vi "Tower_Crane_Balance_Monitor.vi"() -> ()   [LabVIEW 2018]
uses:
  <vilib>/Utility/error.llb/DialogType.ctl
panel:
  out "new picture 4":picture caption="Opertion_Guide"
  out "new picture 3":picture caption="Opertion_Guide"
  out "new picture 2":picture caption="Opertion_Guide"
  out "stanard_section 2":picture caption="配平状态"
  out "X倾斜角度 2":dbl caption="塔身X倾斜角度" format="%#_3g"
  out "Y倾斜角度  2":dbl caption="塔身Y倾斜角度" format="%#_3g"
  out "y轴倾角 2":dbl(knob) scale=0.0..5.0
  out "x轴倾角 2":dbl(knob) scale=0.0..5.0
  out "配平指示1":bool
  out "超声波雷达4":dbl format="%.3f"
  out "超声波雷达4 6":dbl(knob) scale=0.0..10.0
  out "超声波雷达35":dbl format="%.3f"
  out "?":dbl(knob) scale=0.0..10.0
  out "超声波雷达2":dbl format="%.3f"
  out "超声波雷达2":dbl(knob) scale=0.0..10.0
  out "超声波雷达1":dbl format="%.3f"
  out "超声波雷达1":dbl(knob) scale=0.0..10.0
  out "起升高度（m）":dbl caption="起升高度（cm）" format="%#_3g"
  out "变幅长度（m）":dbl format="%#_3g"
  out "风速（m/s）":dbl format="%.3f"
  out "Y倾斜角度":dbl caption="套架Y倾斜角度" format="%#_3g"
  out "X倾斜角度":dbl caption="套架X倾斜角度" format="%#_3g"
  out "回转角度（°）":dbl format="%#_3g"
  out "回转角度":dbl(knob) scale=0.0..10.0
  out "风速":dbl(knob) scale=0.0..10.0
  out "变幅长度":dbl(knob) scale=0.0..140.0
  out "y轴倾角":dbl(knob) scale=0.0..5.0
  out "x轴倾角":dbl(knob) scale=0.0..5.0
  out "起升高度":dbl(slide) caption="顶升高度          (cm)" scale=0.0..180.0
  out "section_connect":picture caption="引进节连接"
  out "rotary_support":picture caption="下回转支座"
  out "stanard_section":picture caption="引进节"
  out "pin_shaft":picture caption="爬爪"
  out "jacking_beam":picture caption="顶升横梁"
  out "new picture":picture caption="Opertion_Guide"
  out "引进滑轮":bool
  out "引进节螺栓4":bool
  out "引进节螺栓3":bool
  out "引进节螺栓2":bool
  out "引进节螺栓1":bool
  out "下回转螺栓4":bool
  out "下回转螺栓3":bool
  out "下回转螺栓2":bool
  out "下回转螺栓1":bool
  out "爬爪右侧":bool
  out "爬爪左侧":bool
  out "横梁右侧":bool
  out "横梁左侧":bool
  in  "倾角串口号 2":refnum<visa-resource-name>
  in  "开始配平":bool
  in  "倾角串口号":refnum<visa-resource-name>
  in  "风速串口号":refnum<visa-resource-name>
  in  "回转编码器":refnum<visa-resource-name>
  in  "变幅编码器":refnum<visa-resource-name>
  in  "高度编码器":refnum<visa-resource-name>
  in  "顶升开关":bool
  in  "滚轮直径D":dbl
  out "倾角读取缓冲区 2":string caption="倾角读取缓冲区"
  out "子字符串 4":string
  out "子字符串 3":string
  out "子字符串 2":string
  out "子字符串":string
  out "数据输出 2":string
  out "esp32的IP地址 2":string
  out "信息来源的端口 2":u16
  in  "清空 2":bool
  out "esp32的IP地址":string
  out "回转圈数":dbl
  out "回转编码器读取缓冲区":string
  out "回转单圈值":dbl
  out "回转编码器错误输出":string
  out "变幅圈数":dbl
  out "小车蝙蝠编码器读取缓冲区":string
  out "变幅单圈值":dbl
  out "回转编码器错误输出1":string
  out "倾角读取缓冲区":string
  out "Wind_Speed_Data":string
  out "风速传感器错误输出":string
  out "操作规范":string
  out "起升圈数":dbl
  out "起升高度编码器读取缓冲区 2":string
  out "起升单圈值":dbl
  out "起升高度编码器数值":dbl
  out "高度编码器错误输出1":string
  out "data out":string
  out "数据输出":string
  out "信息来源的端口":u16
  in  "停止":bool
  in  "清空":bool
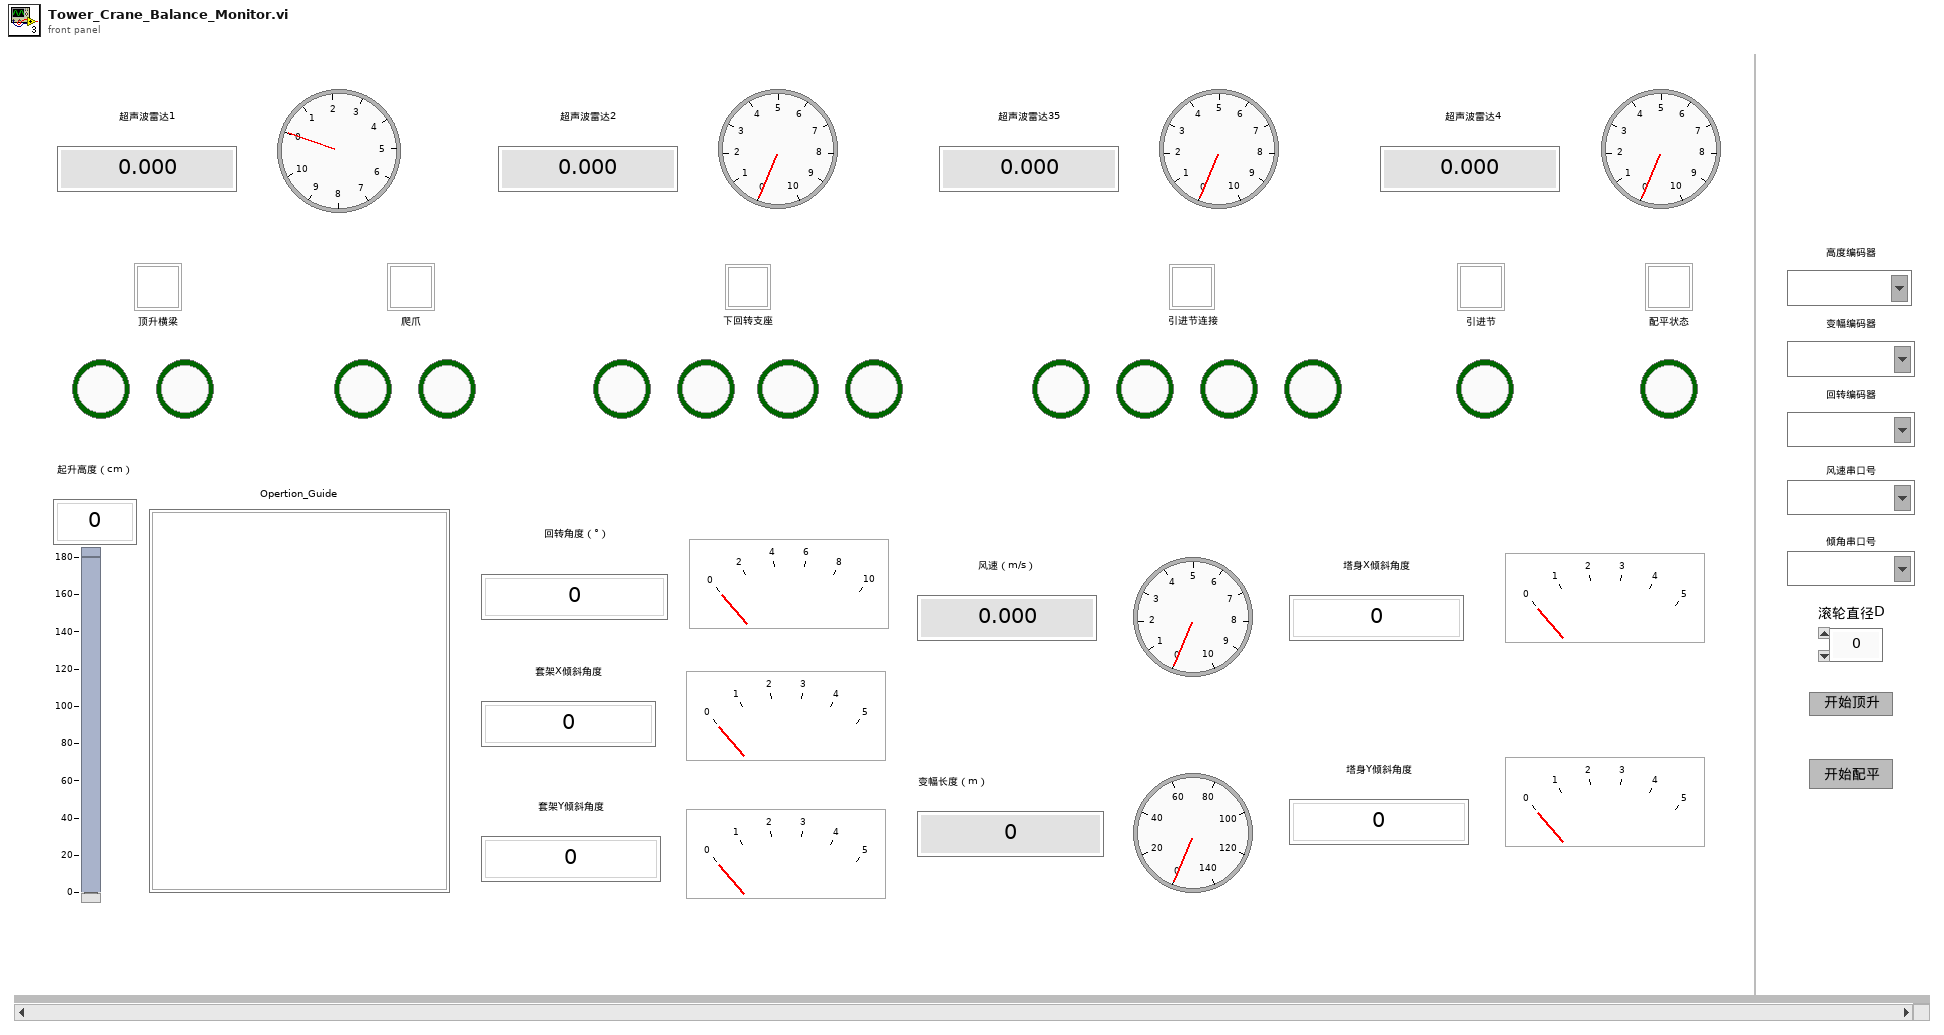
[diagram p1: front panel]
types:
  T1 = typedef "DialogType.ctl" = u16
  T2 = typedef "imagedata.ctl" = cluster{"image type":i32, "image depth":i32, "image":u8[], "mask":u8[], "colors":u32[], "Rectangle":cluster{"left":i16, "top":i16, "right":i16, "bottom":i16}}
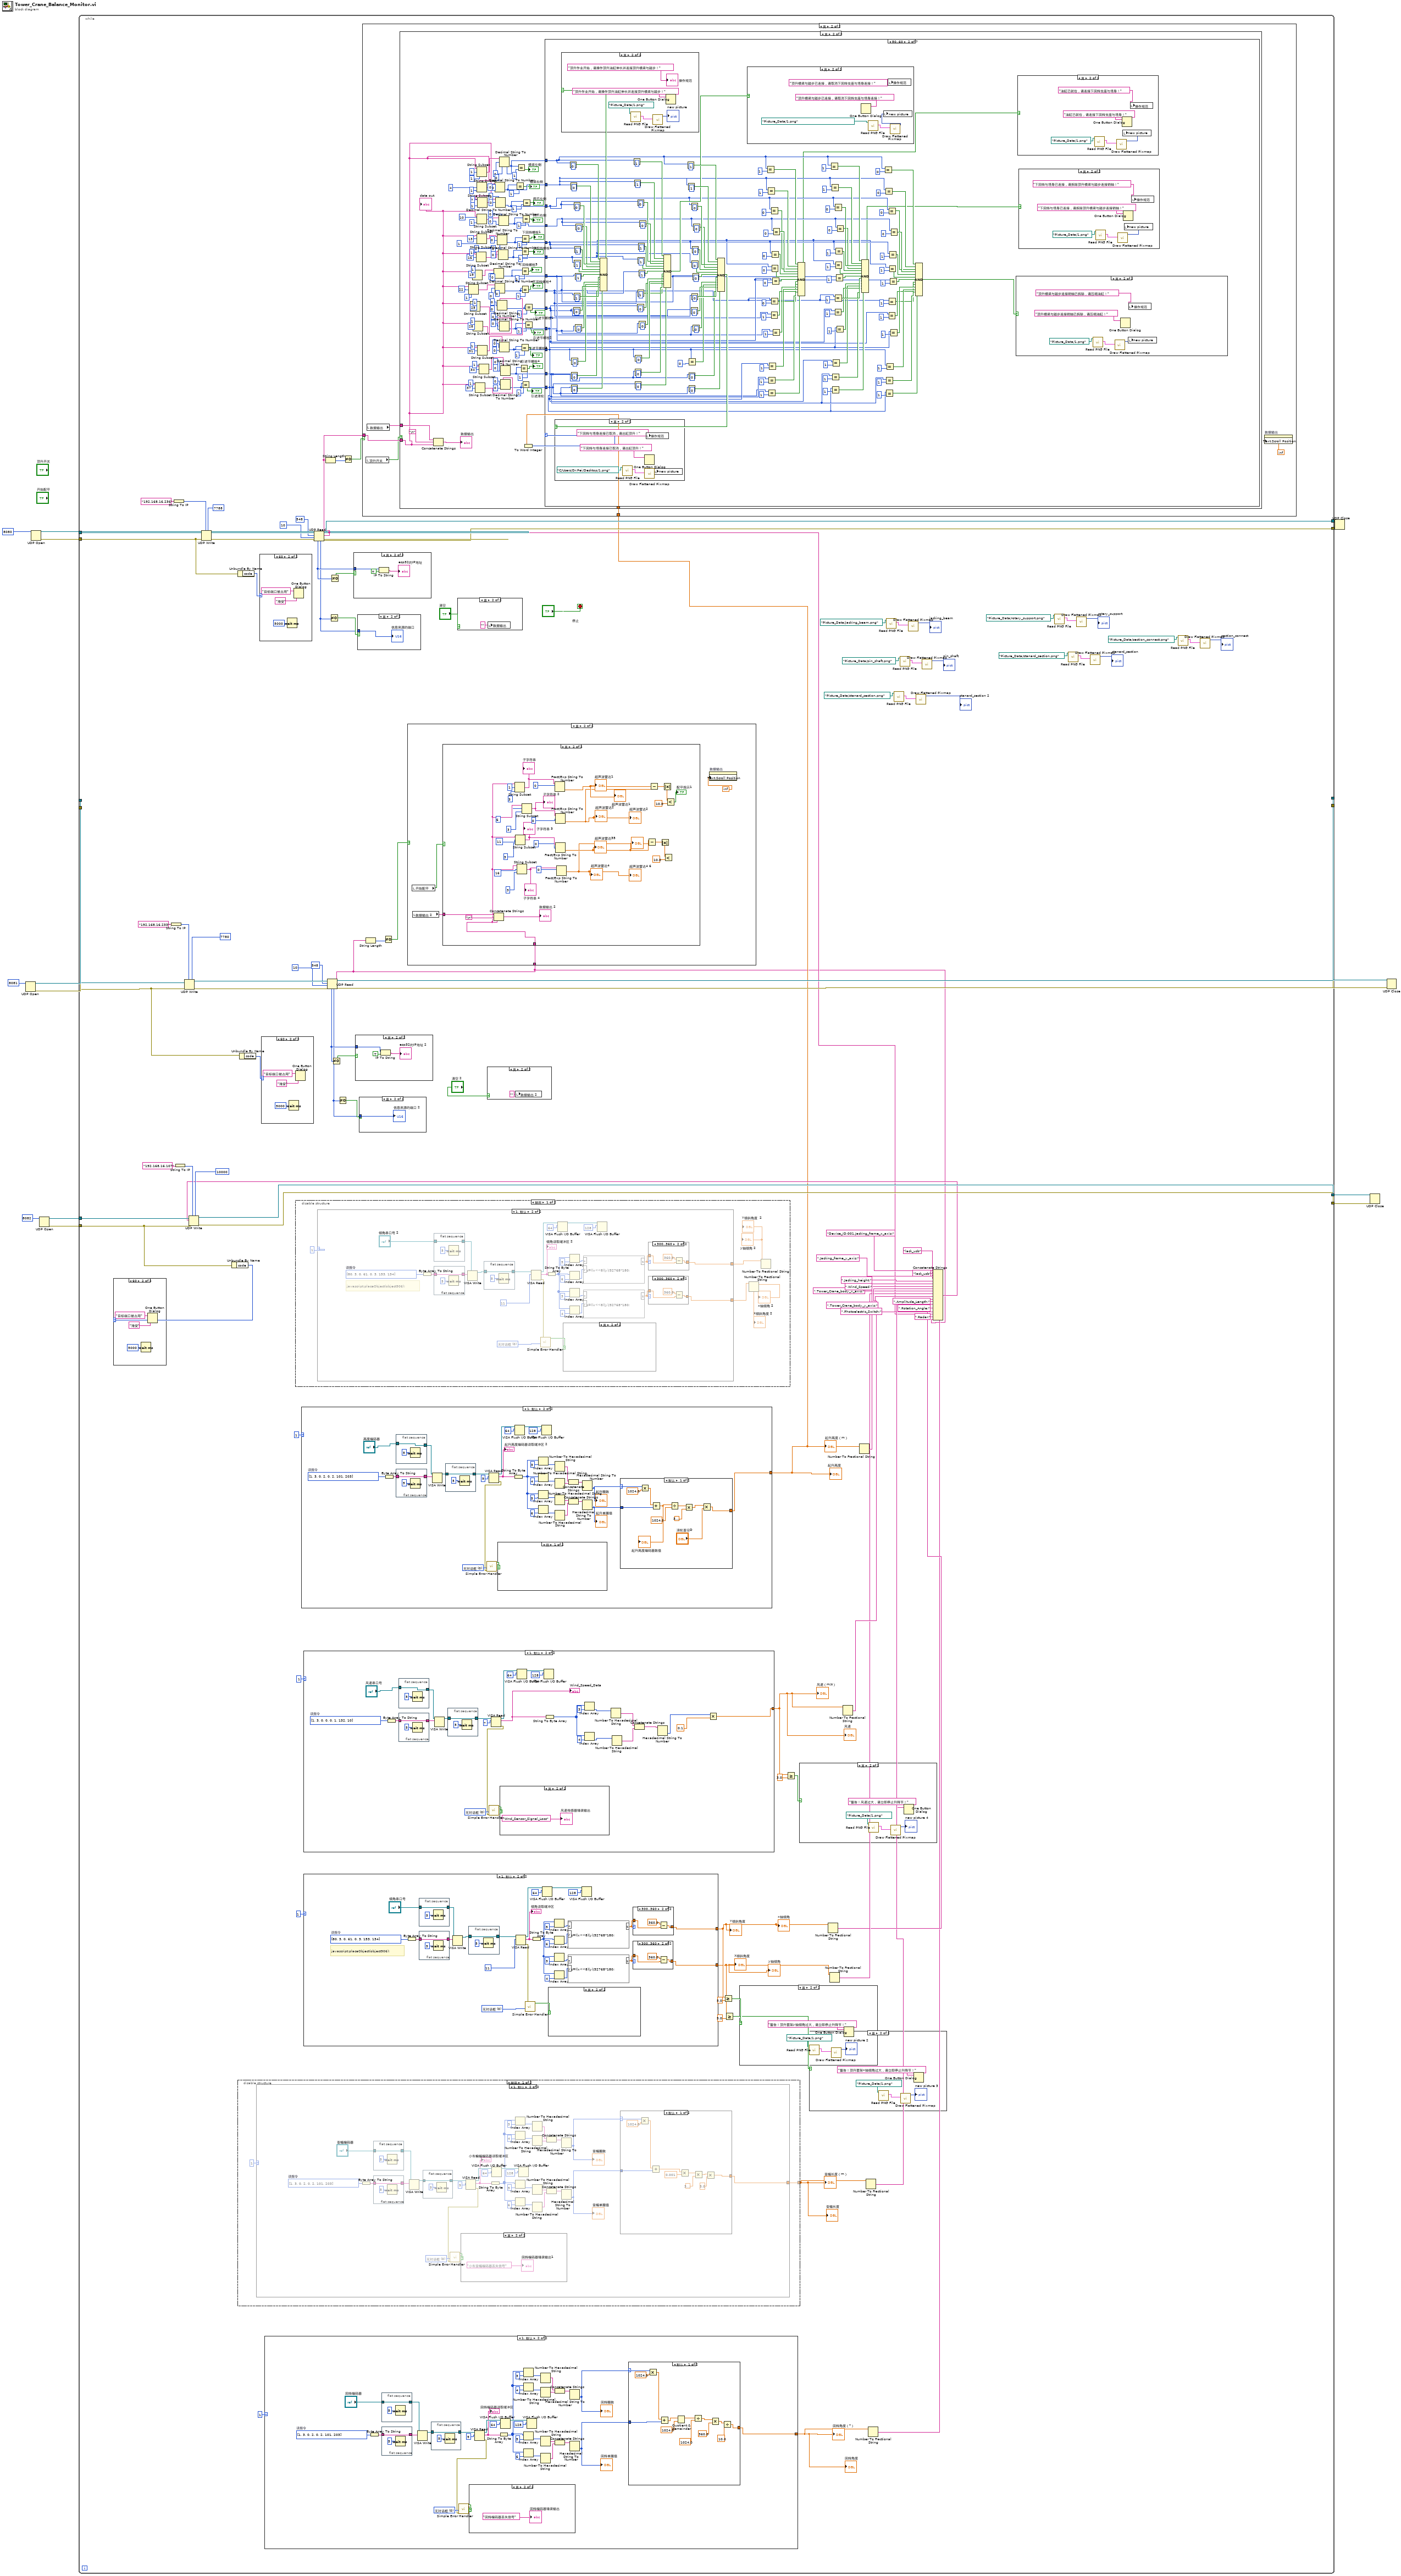
[diagram p0: block diagram]
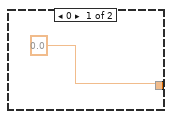
[diagram p2: hidden frame]
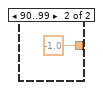
[diagram p4: hidden frame]
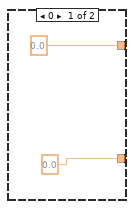
[diagram p9: hidden frame]
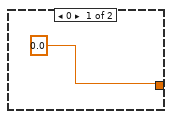
[diagram p14: hidden frame]
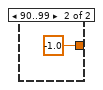
[diagram p16: hidden frame]
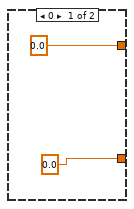
[diagram p17: hidden frame]
diagram:
  n1 = UDP Open(11:u16 8081 ("端口")) -> (port=w9:refnum<k16>, 0:w7:errorcluster)  [unwired: 4 in, 1 out]
  n2 = UDP Open(11:u16 8080 ("端口")) -> (port=w15:refnum<k16>, 0:w14:errorcluster)  [unwired: 4 in, 1 out]
  n3 = UDP Open(11:u16 8082 ("端口")) -> (port=w3:refnum<k16>, 0:w4:errorcluster)  [unwired: 4 in, 1 out]
  n4 = while {
    tunnel: w15 -> [w89]
    tunnel: w14 -> [w84]
    tunnel: [w117] -> w13
    tunnel: [w114] -> w12
    tunnel: w9 -> [w79]
    tunnel: [w77] -> w8
    tunnel: w7 -> [w75]
    tunnel: [w66] -> w6
    tunnel: w4 -> [w58]
    tunnel: w3 -> [w62]
    tunnel: [w57] -> w2
    tunnel: [w56] -> w1
    stop <- "停止" stop-if-true
    n5 = String To IP(1:"192.168.16.233" ("名称")) -> (0:w72:u32)
    n6 = String To IP(1:"192.168.16.236" ("名称")) -> (0:w86:u32)
    n7 = String To IP(1:"192.168.16.107" ("名称")) -> (0:w61:u32)
    n8 = UDP Write(address=w72, port or service name=u16 7780 ("端口或服务名称"), connection ID=w79, 8:w75) -> (error out=w76:errorcluster, 3:w78:refnum<k16>)  [unwired: 2 in]
    n9 = UDP Write(address=w86, port or service name=u16 7788 ("端口或服务名称"), connection ID=w89, 8:w84) -> (error out=w85:errorcluster, 3:w88:refnum<k16>)  [unwired: 2 in]
    n10 = Unbundle By Name(w58) -> ("code"=w59:i32)
    n11 = case shown="60" w59 {
      frame 0, Default {
      }
      frame 60 {
        n12 = Wait (ms)(milliseconds to wait=u32 5000 ("等待时间（毫秒）")) -> ()  [unwired: 1 out]
        n13 = One Button Dialog(message="目标端口被占用" ("消息"), button name ("OK")="难受" ("按钮名称（“确定”）")) -> ()  [unwired: 1 out]
      }
    }
    n14 = disable-structure shown="禁用" {
      disable-tunnel: [w118 _] -> w41
      frame Disabled {
        n15 = case shown="1, 默认" 1 {
          tunnel: [0.0 w126] -> w118
          frame 0 {
          }
          frame 1, Default {
            w124 = T1 0 items=["无对话框", "确定信息", "继续或停止信息", "确定信息＋警告", "继续/停止+警告"] ("type of dialog (OK msg:1)")
            w127 = i32[] [1, 3, 0, 2, 0, 2, 101, 203]  # 读指令
            n16 = Byte Array To String(unsigned byte array=w127) -> (string=w144:string)
            n17 = flat-sequence {
              tunnel: "变幅编码器" -> [w172]
              tunnel: [w172] -> w121
              frame #0 {
                n18 = Wait (ms)(milliseconds to wait=5) -> ()  [unwired: 1 out]
              }
            }
            n19 = flat-sequence {
              tunnel: [w170] -> w143
              tunnel: w144 -> [w170]
              frame #0 {
                n20 = Wait (ms)(milliseconds to wait=5) -> ()  [unwired: 1 out]
              }
            }
            n21 = VISA Write(VISA resource name=w121, write buffer=w143) -> (VISA resource name out=w135:refnum<visa-resource-name>)  [unwired: 1 in, 2 out]
            n22 = flat-sequence {
              tunnel: [w168] -> w136
              tunnel: w135 -> [w168]
              frame #0 {
                n23 = Wait (ms)(milliseconds to wait=5) -> ()  [unwired: 1 out]
              }
            }
            n24 = VISA Read(VISA resource name=w136, byte count=u32 9 ("字节总数")) -> (VISA resource name out=w152:refnum<visa-resource-name>, read buffer=w142:string, error out=w123:errorcluster)  [unwired: 1 in, 1 out]
            "小车蝙蝠编码器读取缓冲区" <- w142
            n25 = call <vilib>:"Simple Error Handler.vi"("type of dialog (OK msg:1)"=w124, "error in (no error)"=w123) -> ("error?"=w125:bool)  [unwired: 3 in, 4 out]
            n26 = case shown="真" w125 {
              frame False {
              }
              frame True {
                "回转编码器错误输出1" <- "小车变幅编码器丢失信号" ("九轴错误输出1")
              }
            }
            n27 = String To Byte Array(string=w142) -> (unsigned byte array=w150:u8[])
            n28 = VISA Flush I/O Buffer(VISA resource name=w152, mask (16)=64) -> (VISA resource name out=w151:refnum<visa-resource-name>)  [unwired: 1 in, 1 out]
            n29 = Index Array ("索引数组")(array=w150, index=3) -> (element=w137:u8)
            n30 = Index Array(array=w150, index=4) -> (element=w141:u8)
            n31 = Index Array ("索引数组")(array=w150, index=5) -> (element=w145:u8)
            n32 = Index Array(array=w150, index=6) -> (element=w149:u8)
            n33 = VISA Flush I/O Buffer(VISA resource name=w151, mask (16)=128) -> ()  [unwired: 1 in, 2 out]
            n34 = Number To Hexadecimal String(2:w137) -> (0:w140:string)  [unwired: 1 in]
            n35 = Number To Hexadecimal String(2:w141) -> (0:w139:string)  [unwired: 1 in]
            n36 = Number To Hexadecimal String(2:w145) -> (0:w148:string)  [unwired: 1 in]
            n37 = Number To Hexadecimal String(2:w149) -> (0:w147:string)  [unwired: 1 in]
            n38 = Concatenate Strings(w140, w139) -> (w138:string)
            n39 = Concatenate Strings(w148, w147) -> (w146:string)
            n40 = Hexadecimal String To Number(string=w138) -> (number=w153:u32)  [unwired: 2 in, 1 out]
            "变幅圈数" <- w153
            n41 = Hexadecimal String To Number(string=w146) -> (number=w154:u32)  [unwired: 2 in, 1 out]
            "变幅单圈值" <- w154
            n42 = case shown="默认" w153 {
              selector: w153 -> [w160 _]
              tunnel: w154 -> [w159 _]
              tunnel: [w158 -1.0] -> w126
              frame Default {
                n43 = Multiply(x=w160, y=1024.0) -> (x*y=w165:dbl)
                n44 = Add(x=w165, y=w159) -> (x+y=w166:dbl)
                n45 = Multiply(x=w166, y=0.001) -> (x*y=w163:dbl)
                n46 = Multiply(x=w163, y=3.141592653589793) -> (x*y=w164:dbl)
                n47 = Multiply(x=w164, y=3.0) -> (x*y=w158:dbl)
              }
              frame 90..99 {
              }
            }
          }
        }
      }
      frame Enabled {
      }
    }
    "变幅长度（m）" <- w41
    "变幅长度" <- w41
    n48 = Unbundle By Name(w84) -> ("code"=w108:i32)
    n49 = Unbundle By Name(w75) -> ("code"=w74:i32)
    n50 = case shown="60" w108 {
      frame 0, Default {
      }
      frame 60 {
        n51 = Wait (ms)(milliseconds to wait=u32 5000 ("等待时间（毫秒）")) -> ()  [unwired: 1 out]
        n52 = One Button Dialog(message="目标端口被占用" ("消息"), button name ("OK")="难受" ("按钮名称（“确定”）")) -> ()  [unwired: 1 out]
      }
    }
    n53 = case shown="60" w74 {
      frame 0, Default {
      }
      frame 60 {
        n54 = Wait (ms)(milliseconds to wait=u32 5000 ("等待时间（毫秒）")) -> ()  [unwired: 1 out]
        n55 = One Button Dialog(message="目标端口被占用" ("消息"), button name ("OK")="难受" ("按钮名称（“确定”）")) -> ()  [unwired: 1 out]
      }
    }
    n56 = case shown="1, 默认" 1 {
      tunnel: [0.0 w240] -> w40
      frame 0 {
      }
      frame 1, Default {
        w238 = T1 0 items=["无对话框", "确定信息", "继续或停止信息", "确定信息＋警告", "继续/停止+警告"] ("type of dialog (OK msg:1)")
        w241 = i32[] [1, 3, 0, 2, 0, 2, 101, 203]  # 读指令
        n57 = Byte Array To String(unsigned byte array=w241) -> (string=w258:string)
        n58 = flat-sequence {
          tunnel: "回转编码器" -> [w288]
          tunnel: [w288] -> w235
          frame #0 {
            n59 = Wait (ms)(milliseconds to wait=5) -> ()  [unwired: 1 out]
          }
        }
        n60 = flat-sequence {
          tunnel: [w286] -> w257
          tunnel: w258 -> [w286]
          frame #0 {
            n61 = Wait (ms)(milliseconds to wait=5) -> ()  [unwired: 1 out]
          }
        }
        n62 = VISA Write(VISA resource name=w235, write buffer=w257) -> (VISA resource name out=w249:refnum<visa-resource-name>)  [unwired: 1 in, 2 out]
        n63 = flat-sequence {
          tunnel: [w284] -> w250
          tunnel: w249 -> [w284]
          frame #0 {
            n64 = Wait (ms)(milliseconds to wait=5) -> ()  [unwired: 1 out]
          }
        }
        n65 = VISA Read(VISA resource name=w250, byte count=u32 9 ("字节总数")) -> (VISA resource name out=w266:refnum<visa-resource-name>, read buffer=w256:string, error out=w237:errorcluster)  [unwired: 1 in, 1 out]
        "回转编码器读取缓冲区" <- w256
        n66 = call <vilib>:"Simple Error Handler.vi"("type of dialog (OK msg:1)"=w238, "error in (no error)"=w237) -> ("error?"=w239:bool)  [unwired: 3 in, 4 out]
        n67 = case shown="真" w239 {
          frame False {
          }
          frame True {
            "回转编码器错误输出" <- "回转编码器丢失信号" ("九轴错误输出1")
          }
        }
        n68 = String To Byte Array(string=w256) -> (unsigned byte array=w264:u8[])
        n69 = VISA Flush I/O Buffer(VISA resource name=w266, mask (16)=64) -> (VISA resource name out=w265:refnum<visa-resource-name>)  [unwired: 1 in, 1 out]
        n70 = Index Array ("索引数组")(array=w264, index=3) -> (element=w251:u8)
        n71 = Index Array(array=w264, index=4) -> (element=w255:u8)
        n72 = Index Array ("索引数组")(array=w264, index=5) -> (element=w259:u8)
        n73 = Index Array(array=w264, index=6) -> (element=w263:u8)
        n74 = VISA Flush I/O Buffer(VISA resource name=w265, mask (16)=128) -> ()  [unwired: 1 in, 2 out]
        n75 = Number To Hexadecimal String(2:w251) -> (0:w254:string)  [unwired: 1 in]
        n76 = Number To Hexadecimal String(2:w255) -> (0:w253:string)  [unwired: 1 in]
        n77 = Number To Hexadecimal String(2:w259) -> (0:w262:string)  [unwired: 1 in]
        n78 = Number To Hexadecimal String(2:w263) -> (0:w261:string)  [unwired: 1 in]
        n79 = Concatenate Strings(w254, w253) -> (w252:string)
        n80 = Concatenate Strings(w262, w261) -> (w260:string)
        n81 = Hexadecimal String To Number(string=w252) -> (number=w267:u32)  [unwired: 2 in, 1 out]
        "回转圈数" <- w267
        n82 = Hexadecimal String To Number(string=w260) -> (number=w268:u32)  [unwired: 2 in, 1 out]
        "回转单圈值" <- w268
        n83 = case shown="默认" w267 {
          selector: w267 -> [w280 _]
          tunnel: w268 -> [w279 _]
          tunnel: [w271 -1.0] -> w240
          frame Default {
            n84 = Multiply(x=w280, y=1024.0) -> (x*y=w282:dbl)
            n85 = Add(x=w282, y=w279) -> (x+y=w278:dbl)
            n86 = Quotient & Remainder(x=w278, y=1024.0) -> (x-y*floor(x/y)=w273:dbl)  [unwired: 1 out]
            n87 = Divide(x=w273, y=1024.0) -> (x/y=w275:dbl)
            n88 = Multiply(x=w275, y=360.0) -> (x*y=w272:dbl)
            n89 = Divide(x=w272, y=10.0) -> (x/y=w271:dbl)
          }
          frame 90..99 {
          }
        }
      }
    }
    "回转角度（°）" <- w40
    "回转角度" <- w40
    n90 = disable-structure shown="禁用" {
      frame Disabled {
        n91 = case shown="1, 默认" 1 {
          tunnel: [0.0 w193] -> w187
          tunnel: [0.0 w199] -> w186
          frame 0 {
          }
          frame 1, Default {
            w196 = T1 0 items=["无对话框", "确定信息", "继续或停止信息", "确定信息＋警告", "继续/停止+警告"] ("type of dialog (OK msg:1)")
            w200 = i32[] [80, 3, 0, 61, 0, 3, 153, 134]  # 读指令
            # "javascript:placeObject(object906);"
            n92 = Byte Array To String(unsigned byte array=w200) -> (string=w212:string)
            n93 = flat-sequence {
              tunnel: "倾角串口号 2" -> [w232]
              tunnel: [w232] -> w194
              frame #0 {
                n94 = Wait (ms)(milliseconds to wait=5) -> ()  [unwired: 1 out]
              }
            }
            n95 = flat-sequence {
              tunnel: [w230] -> w191
              tunnel: w212 -> [w230]
              frame #0 {
                n96 = Wait (ms)(milliseconds to wait=5) -> ()  [unwired: 1 out]
              }
            }
            n97 = VISA Write(VISA resource name=w194, write buffer=w191) -> (VISA resource name out=w208:refnum<visa-resource-name>)  [unwired: 1 in, 2 out]
            n98 = flat-sequence {
              tunnel: w208 -> [w228]
              tunnel: [w228] -> w209
              frame #0 {
                n99 = Wait (ms)(milliseconds to wait=5) -> ()  [unwired: 1 out]
              }
            }
            n100 = VISA Read(VISA resource name=w209, byte count=u32 11 ("字节总数")) -> (VISA resource name out=w216:refnum<visa-resource-name>, read buffer=w192:string, error out=w197:errorcluster)  [unwired: 1 in, 1 out]
            "倾角读取缓冲区 2" <- w192
            n101 = call <vilib>:"Simple Error Handler.vi"("type of dialog (OK msg:1)"=w196, "error in (no error)"=w197) -> ("error?"=w198:bool)  [unwired: 3 in, 4 out]
            n102 = String To Byte Array(string=w192) -> (unsigned byte array=w217:u8[])
            n103 = VISA Flush I/O Buffer(VISA resource name=w216, mask (16)=64) -> (VISA resource name out=w215:refnum<visa-resource-name>)  [unwired: 1 in, 1 out]
            n104 = case shown="真" w198 {
              frame False {
              }
              frame True {
              }
            }
            n105 = Index Array(array=w217, index=5) -> (element=w214:u8)
            n106 = Index Array(array=w217, index=6) -> (element=w213:u8)
            n107 = Index Array(array=w217, index=3) -> (element=w211:u8)
            n108 = Index Array(array=w217, index=4) -> (element=w210:u8)
            n109 = formula code="z=((x<<8)|y)/32768*180;"("x"=w214, "y"=w213) -> ("z"=w219:dbl)
            n110 = formula code="z=((x<<8)|y)/32768*180;"("x"=w211, "y"=w210) -> ("z"=w218:dbl)
            n111 = VISA Flush I/O Buffer(VISA resource name=w215, mask (16)=128) -> ()  [unwired: 1 in, 2 out]
            n112 = case shown="300..360" w219 {
              tunnel: [w224 w226] -> w193
              tunnel: w219 -> [w224 w225]
              frame Default {
              }
              frame 300..360 {
                n113 = Subtract(x=360.0, y=w225) -> (x-y=w226:dbl)
              }
            }
            n114 = case shown="300..360" w218 {
              tunnel: [w220 w222] -> w199
              tunnel: w218 -> [w220 w221]
              frame Default {
              }
              frame 300..360 {
                n115 = Subtract(x=360.0, y=w221) -> (x-y=w222:dbl)
              }
            }
          }
        }
        "X倾斜角度 2" <- w186
        "Y倾斜角度  2" <- w187
        "y轴倾角 2" <- w187
        "x轴倾角 2" <- w186
        n116 = Number To Fractional String(number=w186) -> ()  [unwired: 3 in, 1 out]
        n117 = Number To Fractional String(number=w187) -> ()  [unwired: 3 in, 1 out]
      }
      frame Enabled {
      }
    }
    n118 = case shown="1, 默认" 1 {
      tunnel: [0.0 w376] -> w48
      frame 0 {
      }
      frame 1, Default {
        w374 = T1 0 items=["无对话框", "确定信息", "继续或停止信息", "确定信息＋警告", "继续/停止+警告"] ("type of dialog (OK msg:1)")
        w377 = i32[] [1, 3, 0, 2, 0, 2, 101, 203]  # 读指令
        n119 = Byte Array To String(unsigned byte array=w377) -> (string=w393:string)
        n120 = flat-sequence {
          tunnel: "高度编码器" -> [w422]
          tunnel: [w422] -> w371
          frame #0 {
            n121 = Wait (ms)(milliseconds to wait=5) -> ()  [unwired: 1 out]
          }
        }
        n122 = flat-sequence {
          tunnel: [w420] -> w392
          tunnel: w393 -> [w420]
          frame #0 {
            n123 = Wait (ms)(milliseconds to wait=5) -> ()  [unwired: 1 out]
          }
        }
        n124 = VISA Write(VISA resource name=w371, write buffer=w392) -> (VISA resource name out=w385:refnum<visa-resource-name>)  [unwired: 1 in, 2 out]
        n125 = flat-sequence {
          tunnel: [w418] -> w386
          tunnel: w385 -> [w418]
          frame #0 {
            n126 = Wait (ms)(milliseconds to wait=5) -> ()  [unwired: 1 out]
          }
        }
        n127 = VISA Read(VISA resource name=w386, byte count=u32 9 ("字节总数")) -> (VISA resource name out=w401:refnum<visa-resource-name>, read buffer=w402:string, error out=w373:errorcluster)  [unwired: 1 in, 1 out]
        "起升高度编码器读取缓冲区 2" <- w402
        n128 = call <vilib>:"Simple Error Handler.vi"("type of dialog (OK msg:1)"=w374, "error in (no error)"=w373) -> ("error?"=w375:bool)  [unwired: 3 in, 4 out]
        n129 = case shown="假" w375 {
          frame False {
          }
          frame True {
            "高度编码器错误输出1" <- "起升高度编码器丢失信号" ("九轴错误输出1")
          }
        }
        n130 = String To Byte Array(string=w402) -> (unsigned byte array=w399:u8[])
        n131 = VISA Flush I/O Buffer(VISA resource name=w401, mask (16)=64) -> (VISA resource name out=w400:refnum<visa-resource-name>)  [unwired: 1 in, 1 out]
        n132 = Index Array ("索引数组")(array=w399, index=3) -> (element=w387:u8)
        n133 = Index Array(array=w399, index=4) -> (element=w391:u8)
        n134 = Index Array ("索引数组")(array=w399, index=5) -> (element=w394:u8)
        n135 = Index Array(array=w399, index=6) -> (element=w398:u8)
        n136 = VISA Flush I/O Buffer(VISA resource name=w400, mask (16)=128) -> ()  [unwired: 1 in, 2 out]
        n137 = Number To Hexadecimal String(2:w387) -> (0:w390:string)  [unwired: 1 in]
        n138 = Number To Hexadecimal String(2:w391) -> (0:w389:string)  [unwired: 1 in]
        n139 = Number To Hexadecimal String(2:w394) -> (0:w397:string)  [unwired: 1 in]
        n140 = Number To Hexadecimal String(2:w398) -> (0:w396:string)  [unwired: 1 in]
        n141 = Concatenate Strings(w390, w389) -> (w388:string)
        n142 = Concatenate Strings(w397, w396) -> (w395:string)
        n143 = Hexadecimal String To Number(string=w388) -> (number=w403:u32)  [unwired: 2 in, 1 out]
        "起升圈数" <- w403
        n144 = Hexadecimal String To Number(string=w395) -> (number=w404:u32)  [unwired: 2 in, 1 out]
        "起升单圈值" <- w404
        n145 = case shown="默认" w403 {
          selector: w403 -> [w413 _]
          tunnel: w404 -> [w414 _]
          tunnel: [w406 -1.0] -> w376
          frame Default {
            n146 = Multiply(x=w413, y=1024.0) -> (x*y=w416:dbl)
            n147 = Add(x=w416, y=w414) -> (x+y=w412:dbl)
            "起升高度编码器数值" <- w412
            n148 = Divide(x=w412, y=1024.0) -> (x/y=w410:dbl)
            n149 = Multiply(x=w410, y=3.141592653589793) -> (x*y=w408:dbl)
            n150 = Multiply(x=w408, y="滚轮直径D") -> (x*y=w406:dbl)
          }
          frame 90..99 {
          }
        }
      }
    }
    "起升高度（m）" <- w48
    "起升高度" <- w48
    n151 = case shown="1, 默认" 1 {
      tunnel: [0.0 w298] -> w24
      tunnel: [0.0 w297] -> w22
      frame 0 {
      }
      frame 1, Default {
        w294 = T1 0 items=["无对话框", "确定信息", "继续或停止信息", "确定信息＋警告", "继续/停止+警告"] ("type of dialog (OK msg:1)")
        w299 = i32[] [80, 3, 0, 61, 0, 3, 153, 134]  # 读指令
        # "javascript:placeObject(object906);"
        n152 = Byte Array To String(unsigned byte array=w299) -> (string=w312:string)
        n153 = flat-sequence {
          tunnel: [w333] -> w293
          tunnel: "倾角串口号" -> [w333]
          frame #0 {
            n154 = Wait (ms)(milliseconds to wait=5) -> ()  [unwired: 1 out]
          }
        }
        n155 = flat-sequence {
          tunnel: [w331] -> w313
          tunnel: w312 -> [w331]
          frame #0 {
            n156 = Wait (ms)(milliseconds to wait=5) -> ()  [unwired: 1 out]
          }
        }
        n157 = VISA Write(VISA resource name=w293, write buffer=w313) -> (VISA resource name out=w308:refnum<visa-resource-name>)  [unwired: 1 in, 2 out]
        n158 = flat-sequence {
          tunnel: w308 -> [w329]
          tunnel: [w329] -> w309
          frame #0 {
            n159 = Wait (ms)(milliseconds to wait=5) -> ()  [unwired: 1 out]
          }
        }
        n160 = VISA Read(VISA resource name=w309, byte count=u32 11 ("字节总数")) -> (VISA resource name out=w317:refnum<visa-resource-name>, read buffer=w307:string, error out=w295:errorcluster)  [unwired: 1 in, 1 out]
        "倾角读取缓冲区" <- w307
        n161 = call <vilib>:"Simple Error Handler.vi"("type of dialog (OK msg:1)"=w294, "error in (no error)"=w295) -> ("error?"=w296:bool)  [unwired: 3 in, 4 out]
        n162 = String To Byte Array(string=w307) -> (unsigned byte array=w318:u8[])
        n163 = VISA Flush I/O Buffer(VISA resource name=w317, mask (16)=64) -> (VISA resource name out=w316:refnum<visa-resource-name>)  [unwired: 1 in, 1 out]
        n164 = case shown="真" w296 {
          frame False {
          }
          frame True {
          }
        }
        n165 = Index Array(array=w318, index=5) -> (element=w315:u8)
        n166 = Index Array(array=w318, index=6) -> (element=w314:u8)
        n167 = Index Array(array=w318, index=3) -> (element=w311:u8)
        n168 = Index Array(array=w318, index=4) -> (element=w310:u8)
        n169 = formula code="z=((x<<8)|y)/32768*180;"("x"=w315, "y"=w314) -> ("z"=w320:dbl)
        n170 = formula code="z=((x<<8)|y)/32768*180;"("x"=w311, "y"=w310) -> ("z"=w319:dbl)
        n171 = VISA Flush I/O Buffer(VISA resource name=w316, mask (16)=128) -> ()  [unwired: 1 in, 2 out]
        n172 = case shown="300..360" w320 {
          tunnel: [w325 w327] -> w298
          tunnel: w320 -> [w325 w326]
          frame Default {
          }
          frame 300..360 {
            n173 = Subtract(x=360.0, y=w326) -> (x-y=w327:dbl)
          }
        }
        n174 = case shown="300..360" w319 {
          tunnel: [w321 w323] -> w297
          tunnel: w319 -> [w321 w322]
          frame Default {
          }
          frame 300..360 {
            n175 = Subtract(x=360.0, y=w322) -> (x-y=w323:dbl)
          }
        }
      }
    }
    "X倾斜角度" <- w22
    "Y倾斜角度" <- w24
    "x轴倾角" <- w24
    "y轴倾角" <- w22
    n176 = case shown="1, 默认" 1 {
      tunnel: [u32 0 w337] -> w18
      frame 0 {
      }
      frame 1, Default {
        w351 = T1 0 items=["无对话框", "确定信息", "继续或停止信息", "确定信息＋警告", "继续/停止+警告"] ("type of dialog (OK msg:1)")
        w353 = i32[] [1, 3, 0, 0, 0, 1, 132, 10]  # 读指令
        n177 = Byte Array To String(unsigned byte array=w353) -> (string=w360:string)
        n178 = flat-sequence {
          tunnel: "风速串口号" -> [w368]
          tunnel: [w368] -> w348
          frame #0 {
            n179 = Wait (ms)(milliseconds to wait=5) -> ()  [unwired: 1 out]
          }
        }
        n180 = flat-sequence {
          tunnel: [w366] -> w359
          tunnel: w360 -> [w366]
          frame #0 {
            n181 = Wait (ms)(milliseconds to wait=5) -> ()  [unwired: 1 out]
          }
        }
        n182 = VISA Write(VISA resource name=w348, write buffer=w359) -> (VISA resource name out=w357:refnum<visa-resource-name>)  [unwired: 1 in, 2 out]
        n183 = flat-sequence {
          tunnel: [w364] -> w358
          tunnel: w357 -> [w364]
          frame #0 {
            n184 = Wait (ms)(milliseconds to wait=5) -> ()  [unwired: 1 out]
          }
        }
        n185 = VISA Read(VISA resource name=w358, byte count=u32 7 ("字节总数")) -> (VISA resource name out=w362:refnum<visa-resource-name>, read buffer=w347:string, error out=w350:errorcluster)  [unwired: 1 in, 1 out]
        "Wind_Speed_Data" <- w347
        n186 = call <vilib>:"Simple Error Handler.vi"("type of dialog (OK msg:1)"=w351, "error in (no error)"=w350) -> ("error?"=w352:bool)  [unwired: 3 in, 4 out]
        n187 = case shown="真" w352 {
          frame False {
          }
          frame True {
            "风速传感器错误输出" <- "Wnd_Sensor_Signal_Loss" ("九轴错误输出1")
          }
        }
        n188 = VISA Flush I/O Buffer(VISA resource name=w362, mask (16)=64) -> (VISA resource name out=w361:refnum<visa-resource-name>)  [unwired: 1 in, 1 out]
        n189 = VISA Flush I/O Buffer(VISA resource name=w361, mask (16)=128) -> ()  [unwired: 1 in, 2 out]
        n190 = String To Byte Array(string=w347) -> (unsigned byte array=w346:u8[])
        n191 = Index Array(array=w346, index=3 ("索引")) -> (element=w343:u8)
        n192 = Index Array(array=w346, index=4 ("索引")) -> (element=w342:u8)
        n193 = Number To Hexadecimal String(2:w343) -> (0:w341:string)  [unwired: 1 in]
        n194 = Number To Hexadecimal String(2:w342) -> (0:w340:string)  [unwired: 1 in]
        n195 = Concatenate Strings(w341, w340) -> (w339:string)
        n196 = Hexadecimal String To Number(string=w339) -> (number=w338:u32)  [unwired: 2 in, 1 out]
        n197 = Multiply(x=w338, y=0.1) -> (x*y=w337:dbl)
      }
    }
    "风速" <- w18
    "风速（m/s）" <- w18
    n198 = UDP Read(connection ID=w88, max size (548)=548 ("最大值(548)"), timeout ms (25000)=10 ("超时毫秒(25000)"), 8:w85) -> (data out=w31:string, error out=w117:errorcluster, 3:w114:refnum<k16>, 4:w107:u16, 6:w111:u32)
    n199 = String Length(string=w31) -> (length=w113:i32)
    n200 = UDP Read(connection ID=w78, max size (548)=548 ("最大值(548)"), timeout ms (25000)=10 ("超时毫秒(25000)"), 8:w76) -> (data out=w30:string, error out=w66:errorcluster, 3:w77:refnum<k16>, 4:w67:u16, 6:w68:u32)
    n201 = Not Equal To 0?(x=w107) -> (x != 0?=w109:bool)
    n202 = Not Equal To 0?(x=w111) -> (x != 0?=w110:bool)
    n203 = Not Equal To 0?(x=w68) -> (x != 0?=w80:bool)
    n204 = Not Equal To 0?(x=w67) -> (x != 0?=w81:bool)
    n205 = Not Equal To 0?(x=w113) -> (x != 0?=w112:bool)
    n206 = case shown="真" w110 {
      tunnel: w111 -> [_ w477]
      frame False {
      }
      frame True {
        n207 = IP To String(1:TRUE ("句点符号？(F)"), 2:w477) -> (0:→"esp32的IP地址":string)
      }
    }
    n208 = case shown="真" w80 {
      tunnel: w68 -> [_ w467]
      frame False {
      }
      frame True {
        n209 = IP To String(1:TRUE ("句点符号？(F)"), 2:w467) -> (0:→"esp32的IP地址 2":string)
      }
    }
    n210 = case shown="真" w109 {
      tunnel: w107 -> [_ w474]
      frame False {
      }
      frame True {
        "信息来源的端口" <- w474
      }
    }
    n211 = case shown="真" w81 {
      tunnel: w67 -> [_ w466]
      frame False {
      }
      frame True {
        "信息来源的端口 2" <- w466
      }
    }
    n212 = case shown="真" w112 {
      tunnel: w31 -> [_ w481]
      tunnel: w48 -> [_ w479]
      frame False {
      }
      frame True {
        n213 = local read "顶升开关"() -> (w478:bool)
        n214 = local read "数据输出"() -> (w482:string)
        n215 = case shown="真" w478 {
          tunnel: w482 -> [w485 w594]
          tunnel: w481 -> [w484 w569]
          tunnel: w479 -> [_ w572]
          frame False {
            n216 = Concatenate Strings(w485, w484) -> (w483:string)
            n217 = local write "数据输出"(w483) -> ()
          }
          frame True {
            (unwired) 0 ("默认(0 I32)")
            n218 = Concatenate Strings(w594, "\n", w569) -> (→"数据输出":string)
            n219 = String Subset(string=w569, offset (0)=22 ("偏移量(0)"), length (rest)=1 ("长度（剩余）")) -> (substring=w530:string)
            n220 = String Subset(string=w569, offset (0)=25 ("偏移量(0)"), length (rest)=1 ("长度（剩余）")) -> (substring=w529:string)
            n221 = String Subset(string=w569, offset (0)=19 ("偏移量(0)"), length (rest)=1 ("长度（剩余）")) -> (substring=w531:string)
            n222 = String Subset(string=w569, offset (0)=28 ("偏移量(0)"), length (rest)=1 ("长度（剩余）")) -> (substring=w528:string)
            n223 = String Subset(string=w569, offset (0)=37 ("偏移量(0)"), length (rest)=1 ("长度（剩余）")) -> (substring=w525:string)
            n224 = String Subset(string=w569, offset (0)=16 ("偏移量(0)"), length (rest)=1 ("长度（剩余）")) -> (substring=w547:string)
            n225 = String Subset(string=w569, offset (0)=4 ("偏移量(0)"), length (rest)=1 ("长度（剩余）")) -> (substring=w582:string)
            n226 = String Subset(string=w569, offset (0)=13 ("偏移量(0)"), length (rest)=1 ("长度（剩余）")) -> (substring=w548:string)
            n227 = String Subset(string=w569, offset (0)=1 ("偏移量(0)"), length (rest)=1 ("长度（剩余）")) -> (substring=w584:string)
            n228 = String Subset(string=w569, offset (0)=10 ("偏移量(0)"), length (rest)=1 ("长度（剩余）")) -> (substring=w581:string)
            n229 = String Subset(string=w569, offset (0)=31 ("偏移量(0)"), length (rest)=1 ("长度（剩余）")) -> (substring=w527:string)
            n230 = String Subset(string=w569, offset (0)=7 ("偏移量(0)"), length (rest)=1 ("长度（剩余）")) -> (substring=w583:string)
            n231 = String Subset(string=w569, offset (0)=34 ("偏移量(0)"), length (rest)=1 ("长度（剩余）")) -> (substring=w526:string)
            n232 = Decimal String To Number(string=w531, offset=0 ("偏移量"), default (0L)=0 ("默认(0 I32)")) -> (number=w501:i32)  [unwired: 1 out]
            n233 = Decimal String To Number(string=w582, offset=0 ("偏移量"), default (0L)=0 ("默认(0 I32)")) -> (number=w509:i32)  [unwired: 1 out]
            n234 = Decimal String To Number(string=w530, offset=0 ("偏移量"), default (0L)=0 ("默认(0 I32)")) -> (number=w500:i32)  [unwired: 1 out]
            n235 = Decimal String To Number(string=w583, offset=0 ("偏移量"), default (0L)=0 ("默认(0 I32)")) -> (number=w507:i32)  [unwired: 1 out]
            n236 = Decimal String To Number(string=w548, offset=0 ("偏移量"), default (0L)=0 ("默认(0 I32)")) -> (number=w503:i32)  [unwired: 1 out]
            n237 = Decimal String To Number(string=w529, offset=0 ("偏移量")) -> (number=w499:i32)  [unwired: 1 in, 1 out]
            n238 = Decimal String To Number(string=w547, offset=0 ("偏移量"), default (0L)=0 ("默认(0 I32)")) -> (number=w502:i32)  [unwired: 1 out]
            n239 = Decimal String To Number(string=w581, offset=0 ("偏移量"), default (0L)=0 ("默认(0 I32)")) -> (number=w505:i32)  [unwired: 1 out]
            n240 = Decimal String To Number(string=w584, offset=0 ("偏移量"), default (0L)=0 ("默认(0 I32)")) -> (number=w524:i32)  [unwired: 1 out]
            n241 = Decimal String To Number(string=w528, offset=0 ("偏移量"), default (0L)=0 ("默认(0 I32)")) -> (number=w498:i32)  [unwired: 1 out]
            n242 = Decimal String To Number(string=w527, offset=0 ("偏移量"), default (0L)=0 ("默认(0 I32)")) -> (number=w497:i32)  [unwired: 1 out]
            n243 = Decimal String To Number(string=w526, offset=0 ("偏移量"), default (0L)=0 ("默认(0 I32)")) -> (number=w496:i32)  [unwired: 1 out]
            n244 = Decimal String To Number(string=w525, offset=0 ("偏移量"), default (0L)=0 ("默认(0 I32)")) -> (number=w495:i32)  [unwired: 1 out]
            n245 = Equal?(x=w509, y=1) -> (x = y?=→"横梁右侧":bool)
            n246 = Equal?(x=w524, y=1) -> (x = y?=→"横梁左侧":bool)
            n247 = Equal?(x=w496, y=1) -> (x = y?=→"引进节螺栓4":bool)
            n248 = Equal?(x=w497, y=1) -> (x = y?=→"引进节螺栓3":bool)
            n249 = Equal?(x=w502, y=1) -> (x = y?=→"下回转螺栓2":bool)
            n250 = Equal?(x=w501, y=1) -> (x = y?=→"下回转螺栓3":bool)
            n251 = Equal?(x=w500, y=1) -> (x = y?=→"下回转螺栓4":bool)
            n252 = Equal?(x=w503, y=1) -> (x = y?=→"下回转螺栓1":bool)
            n253 = Equal?(x=w495, y=1) -> (x = y?=→"引进滑轮":bool)
            n254 = Equal?(x=w505, y=1) -> (x = y?=→"爬爪右侧":bool)
            n255 = Equal?(x=w507, y=1) -> (x = y?=→"爬爪左侧":bool)
            n256 = To Word Integer(number=w572) -> (16bit integer=w571:i16)
            n257 = Equal?(x=w498, y=1) -> (x = y?=→"引进节螺栓2":bool)
            n258 = Equal?(x=w499, y=1) -> (x = y?=→"引进节螺栓1":bool)
            n259 = case shown="50..60" w571 {
              tunnel: w524 -> [w610 w725 w940 w1018 w1093 _ w1175]
              tunnel: w509 -> [w609 w724 w941 w1017 w1092 _ w1174]
              tunnel: w507 -> [w608 w723 w939 w1016 w1091 _ w1173]
              tunnel: w505 -> [w607 w722 w938 w1015 w1090 _ w1172]
              tunnel: w503 -> [w606 w721 w937 w1014 w1089 _ w1171]
              tunnel: w502 -> [w605 w720 w936 w1013 w1088 _ w1170]
              tunnel: w501 -> [w604 w719 w935 w1012 w1087 _ w1169]
              tunnel: w500 -> [w603 w718 w934 w1011 w1086 _ w1168]
              tunnel: w499 -> [w602 w717 w933 w1010 w1085 _ w1167]
              tunnel: w498 -> [w601 w710 w932 w1009 w1084 _ w1166]
              tunnel: w497 -> [w600 w716 w931 w1008 w1083 _ w1165]
              tunnel: w496 -> [w599 w715 w930 w1007 w1082 _ w1164]
              tunnel: w495 -> [w598 w714 w929 w1006 w1081 _ w1163]
              frame 25..30, Default {
                n260 = Equal?(x=w610, y=0) -> (x = y?=w688:bool)
                n261 = Equal?(x=w609, y=0) -> (x = y?=w687:bool)
                n262 = Equal?(x=w599, y=0) -> (x = y?=w677:bool)
                n263 = Equal?(x=w598, y=0) -> (x = y?=w676:bool)
                n264 = Equal?(x=w600, y=0) -> (x = y?=w678:bool)
                n265 = Equal?(x=w602, y=0) -> (x = y?=w680:bool)
                n266 = Equal?(x=w608, y=1) -> (x = y?=w686:bool)
                n267 = Equal?(x=w603, y=0) -> (x = y?=w681:bool)
                n268 = Equal?(x=w605, y=0) -> (x = y?=w683:bool)
                n269 = Equal?(x=w606, y=0) -> (x = y?=w684:bool)
                n270 = Equal?(x=w604, y=0) -> (x = y?=w682:bool)
                n271 = Equal?(x=w601, y=0) -> (x = y?=w679:bool)
                n272 = Equal?(x=w607, y=1) -> (x = y?=w685:bool)
                n273 = Compound Arithmetic op=AND ("复合运算")(w688, w687, w686, w685, w684, w683, w682, w681, w680, w679, w678, w677, w676) -> (w597:bool)
                n274 = Equal?(x=w610, y=1) -> (x = y?=w663:bool)
                n275 = Equal?(x=w609, y=1) -> (x = y?=w664:bool)
                n276 = Equal?(x=w599, y=0) -> (x = y?=w674:bool)
                n277 = Equal?(x=w598, y=0) -> (x = y?=w675:bool)
                n278 = Equal?(x=w600, y=0) -> (x = y?=w673:bool)
                n279 = Equal?(x=w602, y=0) -> (x = y?=w671:bool)
                n280 = Equal?(x=w608, y=1) -> (x = y?=w665:bool)
                n281 = Equal?(x=w603, y=0) -> (x = y?=w670:bool)
                n282 = Equal?(x=w605, y=0) -> (x = y?=w668:bool)
                n283 = Equal?(x=w606, y=0) -> (x = y?=w667:bool)
                n284 = Equal?(x=w604, y=0) -> (x = y?=w669:bool)
                n285 = Equal?(x=w601, y=0) -> (x = y?=w672:bool)
                n286 = Equal?(x=w607, y=1) -> (x = y?=w666:bool)
                n287 = Compound Arithmetic op=AND ("复合运算")(w663, w664, w665, w666, w667, w668, w669, w670, w671, w672, w673, w674, w675) -> (w596:bool)
                n288 = Equal?(x=w610, y=1) -> (x = y?=w662:bool)
                n289 = Equal?(x=w609, y=1) -> (x = y?=w661:bool)
                n290 = Equal?(x=w599, y=0) -> (x = y?=w651:bool)
                n291 = Equal?(x=w598, y=0) -> (x = y?=w650:bool)
                n292 = Equal?(x=w600, y=0) -> (x = y?=w652:bool)
                n293 = Equal?(x=w602, y=0) -> (x = y?=w654:bool)
                n294 = Equal?(x=w608, y=0) -> (x = y?=w660:bool)
                n295 = Equal?(x=w603, y=0) -> (x = y?=w655:bool)
                n296 = Equal?(x=w605, y=0) -> (x = y?=w657:bool)
                n297 = Equal?(x=w606, y=0) -> (x = y?=w658:bool)
                n298 = Equal?(x=w604, y=0) -> (x = y?=w656:bool)
                n299 = Equal?(x=w601, y=0) -> (x = y?=w653:bool)
                n300 = Equal?(x=w607, y=0) -> (x = y?=w659:bool)
                n301 = Compound Arithmetic op=AND ("复合运算")(w662, w661, w660, w659, w658, w657, w656, w655, w654, w653, w652, w651, w650) -> (w595:bool)
                n302 = case shown="真" w596 {
                  frame False {
                    n303 = call "Empty Picture"() -> ("empty picture"=w690:picture)
                    n304 = local write "new picture"(w690) -> ()
                    n305 = local write "操作规范"("" ("字符串")) -> ()
                  }
                  frame True {
                    n306 = call <vilib>:"Read PNG File.vi"("path to PNG file"=path "Picture_Data/1.png" ("path to JPEG file")) -> ("image data"=w695:T2)  [unwired: 8 in, 2 out]
                    n307 = call <vilib>:"Draw Flattened Pixmap.vi"("image data"=w695) -> ("new picture"=w691:picture)  [unwired: 8 in]
                    n308 = One Button Dialog(message="顶升横梁与踏步连接销轴已连接，请掀起爬爪！" ("消息")) -> ()  [unwired: 1 in, 1 out]
                    n309 = local write "操作规范"("顶升横梁与踏步连接销轴已连接，请掀起爬爪！" ("字符串")) -> ()
                    n310 = local write "new picture"(w691) -> ()
                  }
                }
                n311 = case shown="真" w597 {
                  frame False {
                    n312 = call "Empty Picture"() -> ("empty picture"=w703:picture)
                    n313 = local write "new picture"(w703) -> ()
                    n314 = local write "操作规范"("" ("字符串")) -> ()
                  }
                  frame True {
                    n315 = call <vilib>:"Read PNG File.vi"("path to PNG file"=path "Picture_Data/1.png" ("path to JPEG file")) -> ("image data"=w709:T2)  [unwired: 8 in, 2 out]
                    n316 = call <vilib>:"Draw Flattened Pixmap.vi"("image data"=w709) -> ("new picture"=w705:picture)  [unwired: 8 in]
                    n317 = One Button Dialog(message="油缸压缩完毕，请连接顶升横梁与踏步连接销轴！" ("消息")) -> ()  [unwired: 1 in, 1 out]
                    n318 = local write "操作规范"("油缸压缩完毕，请连接顶升横梁与踏步连接销轴！" ("字符串")) -> ()
                    n319 = local write "new picture"(w705) -> ()
                  }
                }
                n320 = case shown="真" w595 {
                  frame False {
                    n321 = call "Empty Picture"() -> ("empty picture"=w696:picture)
                    n322 = local write "new picture"(w696) -> ()
                    n323 = local write "操作规范"("" ("字符串")) -> ()
                  }
                  frame True {
                    n324 = call <vilib>:"Read PNG File.vi"("path to PNG file"=path "Picture_Data/1.png" ("path to JPEG file")) -> ("image data"=w702:T2)  [unwired: 8 in, 2 out]
                    n325 = call <vilib>:"Draw Flattened Pixmap.vi"("image data"=w702) -> ("new picture"=w699:picture)  [unwired: 8 in]
                    n326 = local write "操作规范"("爬爪已掀起，请出缸顶升至容纳引进节！" ("字符串")) -> ()
                    n327 = One Button Dialog(message="爬爪已掀起，请出缸顶升至容纳引进节！" ("消息")) -> ()  [unwired: 1 in, 1 out]
                    n328 = local write "new picture"(w699) -> ()
                  }
                }
              }
              frame 50..60 {
                n329 = Equal?(x=w725, y=0) -> (x = y?=w884:bool)
                n330 = Equal?(x=w724, y=0) -> (x = y?=w883:bool)
                n331 = Equal?(x=w715, y=0) -> (x = y?=w873:bool)
                n332 = Equal?(x=w714, y=0) -> (x = y?=w872:bool)
                n333 = Equal?(x=w716, y=0) -> (x = y?=w874:bool)
                n334 = Equal?(x=w717, y=0) -> (x = y?=w876:bool)
                n335 = Equal?(x=w723, y=0) -> (x = y?=w882:bool)
                n336 = Equal?(x=w718, y=1) -> (x = y?=w877:bool)
                n337 = Equal?(x=w720, y=1) -> (x = y?=w879:bool)
                n338 = Equal?(x=w721, y=1) -> (x = y?=w880:bool)
                n339 = Equal?(x=w719, y=1) -> (x = y?=w878:bool)
                n340 = Equal?(x=w710, y=0) -> (x = y?=w875:bool)
                n341 = Equal?(x=w722, y=0) -> (x = y?=w881:bool)
                n342 = Compound Arithmetic op=AND ("复合运算")(w884, w883, w882, w881, w880, w879, w878, w877, w876, w875, w874, w873, w872) -> (w806:bool)
                n343 = case shown="真" w806 {
                  frame False {
                    n344 = call "Empty Picture"() -> ("empty picture"=w921:picture)
                    n345 = local write "new picture"(w921) -> ()
                    n346 = local write "操作规范"("" ("字符串")) -> ()
                  }
                  frame True {
                    n347 = call <vilib>:"Read PNG File.vi"("path to PNG file"=path "Picture_Data/1.png" ("path to JPEG file")) -> ("image data"=w925:T2)  [unwired: 8 in, 2 out]
                    n348 = call <vilib>:"Draw Flattened Pixmap.vi"("image data"=w925) -> ("new picture"=→"new picture":picture)  [unwired: 8 in]
                    n349 = One Button Dialog(message="顶升作业开始，请操作顶升油缸伸长并连接顶升横梁与踏步！" ("消息")) -> ()  [unwired: 1 in, 1 out]
                    "操作规范" <- "顶升作业开始，请操作顶升油缸伸长并连接顶升横梁与踏步！" ("字符串")
                  }
                }
                n350 = Equal?(x=w725, y=1) -> (x = y?=w859:bool)
                n351 = Equal?(x=w724, y=1) -> (x = y?=w860:bool)
                n352 = Equal?(x=w715, y=0) -> (x = y?=w870:bool)
                n353 = Equal?(x=w714, y=0) -> (x = y?=w871:bool)
                n354 = Equal?(x=w716, y=0) -> (x = y?=w869:bool)
                n355 = Equal?(x=w717, y=0) -> (x = y?=w867:bool)
                n356 = Equal?(x=w723, y=0) -> (x = y?=w861:bool)
                n357 = Equal?(x=w718, y=1) -> (x = y?=w866:bool)
                n358 = Equal?(x=w720, y=1) -> (x = y?=w864:bool)
                n359 = Equal?(x=w721, y=1) -> (x = y?=w863:bool)
                n360 = Equal?(x=w719, y=1) -> (x = y?=w865:bool)
                n361 = Equal?(x=w710, y=0) -> (x = y?=w868:bool)
                n362 = Equal?(x=w722, y=0) -> (x = y?=w862:bool)
                n363 = Compound Arithmetic op=AND ("复合运算")(w859, w860, w861, w862, w863, w864, w865, w866, w867, w868, w869, w870, w871) -> (w726:bool)
                n364 = Equal?(x=w725, y=1) -> (x = y?=w858:bool)
                n365 = Equal?(x=w724, y=1) -> (x = y?=w857:bool)
                n366 = Equal?(x=w715, y=0) -> (x = y?=w847:bool)
                n367 = Equal?(x=w714, y=0) -> (x = y?=w846:bool)
                n368 = Equal?(x=w716, y=0) -> (x = y?=w848:bool)
                n369 = Equal?(x=w717, y=0) -> (x = y?=w850:bool)
                n370 = Equal?(x=w723, y=0) -> (x = y?=w856:bool)
                n371 = Equal?(x=w718, y=0) -> (x = y?=w851:bool)
                n372 = Equal?(x=w720, y=0) -> (x = y?=w853:bool)
                n373 = Equal?(x=w721, y=0) -> (x = y?=w854:bool)
                n374 = Equal?(x=w719, y=0) -> (x = y?=w852:bool)
                n375 = Equal?(x=w710, y=0) -> (x = y?=w849:bool)
                n376 = Equal?(x=w722, y=0) -> (x = y?=w855:bool)
                n377 = Compound Arithmetic op=AND ("复合运算")(w858, w857, w856, w855, w854, w853, w852, w851, w850, w849, w848, w847, w846) -> (w805:bool)
                n378 = case shown="真" w805 {
                  frame False {
                    n379 = call "Empty Picture"() -> ("empty picture"=w907:picture)
                    n380 = local write "new picture"(w907) -> ()
                    n381 = local write "操作规范"("" ("字符串")) -> ()
                  }
                  frame True {
                    n382 = call <vilib>:"Read PNG File.vi"("path to PNG file"=path "C:/Users/Dr.Pei/Desktop/1.png" ("path to JPEG file")) -> ("image data"=w911:T2)  [unwired: 8 in, 2 out]
                    n383 = One Button Dialog(message="下回转与塔身连接已取消，请出缸顶升！" ("消息")) -> ()  [unwired: 1 in, 1 out]
                    n384 = call <vilib>:"Draw Flattened Pixmap.vi"("image data"=w911) -> ("new picture"=w910:picture)  [unwired: 8 in]
                    n385 = local write "操作规范"("下回转与塔身连接已取消，请出缸顶升！" ("字符串")) -> ()
                    n386 = local write "new picture"(w910) -> ()
                  }
                }
                n387 = case shown="真" w726 {
                  frame False {
                    n388 = call "Empty Picture"() -> ("empty picture"=w914:picture)
                    n389 = local write "操作规范"("" ("字符串")) -> ()
                    n390 = local write "new picture"(w914) -> ()
                  }
                  frame True {
                    n391 = One Button Dialog(message="顶升横梁与踏步已连接，请取消下回转支座与塔身连接！" ("消息")) -> ()  [unwired: 1 in, 1 out]
                    n392 = call <vilib>:"Read PNG File.vi"("path to PNG file"=path "Picture_Data/1.png" ("path to JPEG file")) -> ("image data"=w918:T2)  [unwired: 8 in, 2 out]
                    n393 = local write "操作规范"("顶升横梁与踏步已连接，请取消下回转支座与塔身连接！" ("字符串")) -> ()
                    n394 = call <vilib>:"Draw Flattened Pixmap.vi"("image data"=w918) -> ("new picture"=w917:picture)  [unwired: 8 in]
                    n395 = local write "new picture"(w917) -> ()
                  }
                }
                n396 = Equal?(x=w725, y=1) -> (x = y?=w727:bool)
                n397 = Equal?(x=w724, y=1) -> (x = y?=w728:bool)
                n398 = Equal?(x=w715, y=1) -> (x = y?=w738:bool)
                n399 = Equal?(x=w714, y=1) -> (x = y?=w739:bool)
                n400 = Equal?(x=w716, y=1) -> (x = y?=w737:bool)
                n401 = Equal?(x=w717, y=1) -> (x = y?=w735:bool)
                n402 = Equal?(x=w723, y=0) -> (x = y?=w729:bool)
                n403 = Equal?(x=w718, y=0) -> (x = y?=w734:bool)
                n404 = Equal?(x=w720, y=0) -> (x = y?=w732:bool)
                n405 = Equal?(x=w721, y=0) -> (x = y?=w731:bool)
                n406 = Equal?(x=w719, y=0) -> (x = y?=w733:bool)
                n407 = Equal?(x=w710, y=1) -> (x = y?=w736:bool)
                n408 = Equal?(x=w722, y=0) -> (x = y?=w730:bool)
                n409 = Compound Arithmetic op=AND ("复合运算")(w727, w728, w729, w730, w731, w732, w733, w734, w735, w736, w737, w738, w739) -> (w713:bool)
                n410 = Equal?(x=w725, y=1) -> (x = y?=w752:bool)
                n411 = Equal?(x=w724, y=1) -> (x = y?=w751:bool)
                n412 = Equal?(x=w715, y=1) -> (x = y?=w741:bool)
                n413 = Equal?(x=w714, y=1) -> (x = y?=w740:bool)
                n414 = Equal?(x=w716, y=1) -> (x = y?=w742:bool)
                n415 = Equal?(x=w717, y=1) -> (x = y?=w744:bool)
                n416 = Equal?(x=w723, y=0) -> (x = y?=w750:bool)
                n417 = Equal?(x=w718, y=1) -> (x = y?=w745:bool)
                n418 = Equal?(x=w720, y=1) -> (x = y?=w747:bool)
                n419 = Equal?(x=w721, y=1) -> (x = y?=w748:bool)
                n420 = Equal?(x=w719, y=1) -> (x = y?=w746:bool)
                n421 = Equal?(x=w710, y=1) -> (x = y?=w743:bool)
                n422 = Equal?(x=w722, y=0) -> (x = y?=w749:bool)
                n423 = Compound Arithmetic op=AND ("复合运算")(w752, w751, w750, w749, w748, w747, w746, w745, w744, w743, w742, w741, w740) -> (w712:bool)
                n424 = Equal?(x=w725, y=0) -> (x = y?=w753:bool)
                n425 = Equal?(x=w724, y=0) -> (x = y?=w754:bool)
                n426 = Equal?(x=w715, y=1) -> (x = y?=w764:bool)
                n427 = Equal?(x=w714, y=1) -> (x = y?=w765:bool)
                n428 = Equal?(x=w716, y=1) -> (x = y?=w763:bool)
                n429 = Equal?(x=w717, y=1) -> (x = y?=w761:bool)
                n430 = Equal?(x=w723, y=0) -> (x = y?=w755:bool)
                n431 = Equal?(x=w718, y=1) -> (x = y?=w760:bool)
                n432 = Equal?(x=w720, y=1) -> (x = y?=w758:bool)
                n433 = Equal?(x=w721, y=1) -> (x = y?=w757:bool)
                n434 = Equal?(x=w719, y=1) -> (x = y?=w759:bool)
                n435 = Equal?(x=w710, y=1) -> (x = y?=w762:bool)
                n436 = Equal?(x=w722, y=0) -> (x = y?=w756:bool)
                n437 = Compound Arithmetic op=AND ("复合运算")(w753, w754, w755, w756, w757, w758, w759, w760, w761, w762, w763, w764, w765) -> (w711:bool)
                n438 = case shown="真" w711 {
                  frame False {
                    n439 = call "Empty Picture"() -> ("empty picture"=w885:picture)
                    n440 = local write "new picture"(w885) -> ()
                    n441 = local write "操作规范"("" ("字符串")) -> ()
                  }
                  frame True {
                    n442 = call <vilib>:"Read PNG File.vi"("path to PNG file"=path "Picture_Data/1.png" ("path to JPEG file")) -> ("image data"=w891:T2)  [unwired: 8 in, 2 out]
                    n443 = call <vilib>:"Draw Flattened Pixmap.vi"("image data"=w891) -> ("new picture"=w887:picture)  [unwired: 8 in]
                    n444 = One Button Dialog(message="顶升横梁与踏步连接销轴已拆除，请压缩油缸！" ("消息")) -> ()  [unwired: 1 in, 1 out]
                    n445 = local write "new picture"(w887) -> ()
                    n446 = local write "操作规范"("顶升横梁与踏步连接销轴已拆除，请压缩油缸！" ("字符串")) -> ()
                  }
                }
                n447 = case shown="真" w713 {
                  frame False {
                    n448 = call "Empty Picture"() -> ("empty picture"=w899:picture)
                    n449 = local write "new picture"(w899) -> ()
                    n450 = local write "操作规范"("" ("字符串")) -> ()
                  }
                  frame True {
                    n451 = call <vilib>:"Read PNG File.vi"("path to PNG file"=path "Picture_Data/1.png" ("path to JPEG file")) -> ("image data"=w905:T2)  [unwired: 8 in, 2 out]
                    n452 = call <vilib>:"Draw Flattened Pixmap.vi"("image data"=w905) -> ("new picture"=w901:picture)  [unwired: 8 in]
                    n453 = One Button Dialog(message="油缸已就位，请连接下回转支座与塔身！" ("消息")) -> ()  [unwired: 1 in, 1 out]
                    n454 = local write "new picture"(w901) -> ()
                    n455 = local write "操作规范"("油缸已就位，请连接下回转支座与塔身！" ("字符串")) -> ()
                  }
                }
                n456 = case shown="真" w712 {
                  frame False {
                    n457 = call "Empty Picture"() -> ("empty picture"=w892:picture)
                    n458 = local write "new picture"(w892) -> ()
                    n459 = local write "操作规范"("" ("字符串")) -> ()
                  }
                  frame True {
                    n460 = call <vilib>:"Read PNG File.vi"("path to PNG file"=path "Picture_Data/1.png" ("path to JPEG file")) -> ("image data"=w898:T2)  [unwired: 8 in, 2 out]
                    n461 = call <vilib>:"Draw Flattened Pixmap.vi"("image data"=w898) -> ("new picture"=w894:picture)  [unwired: 8 in]
                    n462 = One Button Dialog(message="下回转与塔身已连接，请拆除顶升横梁与踏步连接销轴！" ("消息")) -> ()  [unwired: 1 in, 1 out]
                    n463 = local write "new picture"(w894) -> ()
                    n464 = local write "操作规范"("下回转与塔身已连接，请拆除顶升横梁与踏步连接销轴！" ("字符串")) -> ()
                  }
                }
              }
              frame 158..168 {
                n465 = Equal?(x=w940, y=1) -> (x = y?=w993:bool)
                n466 = Equal?(x=w941, y=1) -> (x = y?=w992:bool)
                n467 = Equal?(x=w930, y=0) -> (x = y?=w982:bool)
                n468 = Equal?(x=w929, y=0) -> (x = y?=w981:bool)
                n469 = Equal?(x=w931, y=0) -> (x = y?=w983:bool)
                n470 = Equal?(x=w933, y=0) -> (x = y?=w985:bool)
                n471 = Equal?(x=w939, y=0) -> (x = y?=w991:bool)
                n472 = Equal?(x=w934, y=0) -> (x = y?=w986:bool)
                n473 = Equal?(x=w936, y=0) -> (x = y?=w988:bool)
                n474 = Equal?(x=w937, y=0) -> (x = y?=w989:bool)
                n475 = Equal?(x=w935, y=0) -> (x = y?=w987:bool)
                n476 = Equal?(x=w932, y=0) -> (x = y?=w984:bool)
                n477 = Equal?(x=w938, y=0) -> (x = y?=w990:bool)
                n478 = Compound Arithmetic op=AND ("复合运算")(w993, w992, w991, w990, w989, w988, w987, w986, w985, w984, w983, w982, w981) -> (w928:bool)
                n479 = Equal?(x=w940, y=1) -> (x = y?=w968:bool)
                n480 = Equal?(x=w941, y=1) -> (x = y?=w969:bool)
                n481 = Equal?(x=w930, y=0) -> (x = y?=w979:bool)
                n482 = Equal?(x=w929, y=0) -> (x = y?=w980:bool)
                n483 = Equal?(x=w931, y=0) -> (x = y?=w978:bool)
                n484 = Equal?(x=w933, y=0) -> (x = y?=w976:bool)
                n485 = Equal?(x=w939, y=1) -> (x = y?=w970:bool)
                n486 = Equal?(x=w934, y=0) -> (x = y?=w975:bool)
                n487 = Equal?(x=w936, y=0) -> (x = y?=w973:bool)
                n488 = Equal?(x=w937, y=0) -> (x = y?=w972:bool)
                n489 = Equal?(x=w935, y=0) -> (x = y?=w974:bool)
                n490 = Equal?(x=w932, y=0) -> (x = y?=w977:bool)
                n491 = Equal?(x=w938, y=1) -> (x = y?=w971:bool)
                n492 = Compound Arithmetic op=AND ("复合运算")(w968, w969, w970, w971, w972, w973, w974, w975, w976, w977, w978, w979, w980) -> (w927:bool)
                n493 = case shown="真" w928 {
                  frame False {
                    (unwired) "" ("字符串")
                    n494 = call "Empty Picture"() -> ()  [unwired: 1 out]
                  }
                  frame True {
                    n495 = call <vilib>:"Read PNG File.vi"("path to PNG file"=path "Picture_Data/1.png" ("path to JPEG file")) -> ("image data"=w1003:T2)  [unwired: 8 in, 2 out]
                    n496 = local write "操作规范"("顶升油缸已到位，请压下爬爪！" ("字符串")) -> ()
                    n497 = call <vilib>:"Draw Flattened Pixmap.vi"("image data"=w1003) -> ("new picture"=w999:picture)  [unwired: 8 in]
                    n498 = One Button Dialog(message="顶升油缸已到位，请压下爬爪！" ("消息")) -> ()  [unwired: 1 in, 1 out]
                    n499 = local write "new picture"(w999) -> ()
                  }
                }
                n500 = case shown="真" w927 {
                  frame False {
                    (unwired) "" ("字符串")
                    n501 = call "Empty Picture"() -> ()  [unwired: 1 out]
                  }
                  frame True {
                    n502 = call <vilib>:"Read PNG File.vi"("path to PNG file"=path "Picture_Data/1.png" ("path to JPEG file")) -> ("image data"=w998:T2)  [unwired: 8 in, 2 out]
                    n503 = local write "操作规范"("爬爪已就位，请压缩油缸！" ("字符串")) -> ()
                    n504 = call <vilib>:"Draw Flattened Pixmap.vi"("image data"=w998) -> ("new picture"=w994:picture)  [unwired: 8 in]
                    n505 = One Button Dialog(message="爬爪已就位，请压缩油缸！" ("消息")) -> ()  [unwired: 1 in, 1 out]
                    n506 = local write "new picture"(w994) -> ()
                  }
                }
              }
              frame 150..155 {
                n507 = Equal?(x=w1018, y=1) -> (x = y?=w1070:bool)
                n508 = Equal?(x=w1017, y=1) -> (x = y?=w1069:bool)
                n509 = Equal?(x=w1007, y=0) -> (x = y?=w1059:bool)
                n510 = Equal?(x=w1006, y=0) -> (x = y?=w1058:bool)
                n511 = Equal?(x=w1008, y=0) -> (x = y?=w1060:bool)
                n512 = Equal?(x=w1010, y=0) -> (x = y?=w1062:bool)
                n513 = Equal?(x=w1016, y=1) -> (x = y?=w1068:bool)
                n514 = Equal?(x=w1011, y=0) -> (x = y?=w1063:bool)
                n515 = Equal?(x=w1013, y=0) -> (x = y?=w1065:bool)
                n516 = Equal?(x=w1014, y=0) -> (x = y?=w1066:bool)
                n517 = Equal?(x=w1012, y=0) -> (x = y?=w1064:bool)
                n518 = Equal?(x=w1009, y=0) -> (x = y?=w1061:bool)
                n519 = Equal?(x=w1015, y=1) -> (x = y?=w1067:bool)
                n520 = Compound Arithmetic op=AND ("复合运算")(w1070, w1069, w1068, w1067, w1066, w1065, w1064, w1063, w1062, w1061, w1060, w1059, w1058) -> (w1005:bool)
                n521 = Equal?(x=w1018, y=0) -> (x = y?=w1045:bool)
                n522 = Equal?(x=w1017, y=0) -> (x = y?=w1046:bool)
                n523 = Equal?(x=w1007, y=0) -> (x = y?=w1056:bool)
                n524 = Equal?(x=w1006, y=0) -> (x = y?=w1057:bool)
                n525 = Equal?(x=w1008, y=0) -> (x = y?=w1055:bool)
                n526 = Equal?(x=w1010, y=0) -> (x = y?=w1053:bool)
                n527 = Equal?(x=w1016, y=1) -> (x = y?=w1047:bool)
                n528 = Equal?(x=w1011, y=0) -> (x = y?=w1052:bool)
                n529 = Equal?(x=w1013, y=0) -> (x = y?=w1050:bool)
                n530 = Equal?(x=w1014, y=0) -> (x = y?=w1049:bool)
                n531 = Equal?(x=w1012, y=0) -> (x = y?=w1051:bool)
                n532 = Equal?(x=w1009, y=0) -> (x = y?=w1054:bool)
                n533 = Equal?(x=w1015, y=1) -> (x = y?=w1048:bool)
                n534 = Compound Arithmetic op=AND ("复合运算")(w1045, w1046, w1047, w1048, w1049, w1050, w1051, w1052, w1053, w1054, w1055, w1056, w1057) -> (w1004:bool)
                n535 = case shown="真" w1004 {
                  frame False {
                    (unwired) "" ("字符串")
                    n536 = call "Empty Picture"() -> ()  [unwired: 1 out]
                  }
                  frame True {
                    n537 = call <vilib>:"Read PNG File.vi"("path to PNG file"=path "Picture_Data/1.png" ("path to JPEG file")) -> ("image data"=w1075:T2)  [unwired: 8 in, 2 out]
                    n538 = call <vilib>:"Draw Flattened Pixmap.vi"("image data"=w1075) -> ("new picture"=w1071:picture)  [unwired: 8 in]
                    n539 = One Button Dialog(message="顶升横梁与踏步连接销轴已拆除，请压缩油缸！" ("消息")) -> ()  [unwired: 1 in, 1 out]
                    n540 = local write "操作规范"("顶升横梁与踏步连接销轴已拆除，请压缩油缸！" ("字符串")) -> ()
                    n541 = local write "new picture"(w1071) -> ()
                  }
                }
                n542 = case shown="真" w1005 {
                  frame False {
                    (unwired) "" ("字符串")
                    n543 = call "Empty Picture"() -> ()  [unwired: 1 out]
                  }
                  frame True {
                    n544 = call <vilib>:"Read PNG File.vi"("path to PNG file"=path "Picture_Data/1.png" ("path to JPEG file")) -> ("image data"=w1080:T2)  [unwired: 8 in, 2 out]
                    n545 = call <vilib>:"Draw Flattened Pixmap.vi"("image data"=w1080) -> ("new picture"=w1076:picture)  [unwired: 8 in]
                    n546 = One Button Dialog(message="油缸已回缩就位，请拆除顶升横梁与踏步连接销轴！" ("消息")) -> ()  [unwired: 1 in, 1 out]
                    n547 = local write "操作规范"("油缸已回缩就位，请拆除顶升横梁与踏步连接销轴！" ("字符串")) -> ()
                    n548 = local write "new picture"(w1076) -> ()
                  }
                }
              }
              frame 120..130 {
                n549 = Equal?(x=w1093, y=1) -> (x = y?=w1147:bool)
                n550 = Equal?(x=w1092, y=1) -> (x = y?=w1146:bool)
                n551 = Equal?(x=w1082, y=0) -> (x = y?=w1136:bool)
                n552 = Equal?(x=w1081, y=0) -> (x = y?=w1135:bool)
                n553 = Equal?(x=w1083, y=0) -> (x = y?=w1137:bool)
                n554 = Equal?(x=w1085, y=0) -> (x = y?=w1139:bool)
                n555 = Equal?(x=w1091, y=0) -> (x = y?=w1145:bool)
                n556 = Equal?(x=w1086, y=0) -> (x = y?=w1140:bool)
                n557 = Equal?(x=w1088, y=0) -> (x = y?=w1142:bool)
                n558 = Equal?(x=w1089, y=0) -> (x = y?=w1143:bool)
                n559 = Equal?(x=w1087, y=0) -> (x = y?=w1141:bool)
                n560 = Equal?(x=w1084, y=0) -> (x = y?=w1138:bool)
                n561 = Equal?(x=w1090, y=0) -> (x = y?=w1144:bool)
                n562 = Compound Arithmetic op=AND ("复合运算")(w1147, w1146, w1145, w1144, w1143, w1142, w1141, w1140, w1139, w1138, w1137, w1136, w1135) -> (w1095:bool)
                n563 = Equal?(x=w1093, y=1) -> (x = y?=w1122:bool)
                n564 = Equal?(x=w1092, y=1) -> (x = y?=w1123:bool)
                n565 = Equal?(x=w1082, y=0) -> (x = y?=w1133:bool)
                n566 = Equal?(x=w1081, y=1) -> (x = y?=w1134:bool)
                n567 = Equal?(x=w1083, y=0) -> (x = y?=w1132:bool)
                n568 = Equal?(x=w1085, y=0) -> (x = y?=w1130:bool)
                n569 = Equal?(x=w1091, y=0) -> (x = y?=w1124:bool)
                n570 = Equal?(x=w1086, y=0) -> (x = y?=w1129:bool)
                n571 = Equal?(x=w1088, y=0) -> (x = y?=w1127:bool)
                n572 = Equal?(x=w1089, y=0) -> (x = y?=w1126:bool)
                n573 = Equal?(x=w1087, y=0) -> (x = y?=w1128:bool)
                n574 = Equal?(x=w1084, y=0) -> (x = y?=w1131:bool)
                n575 = Equal?(x=w1090, y=0) -> (x = y?=w1125:bool)
                n576 = Compound Arithmetic op=AND ("复合运算")(w1122, w1123, w1124, w1125, w1126, w1127, w1128, w1129, w1130, w1131, w1132, w1133, w1134) -> (w1094:bool)
                n577 = case shown="真" w1095 {
                  frame False {
                    n578 = call "Empty Picture"() -> ("empty picture"=w1156:picture)
                    n579 = local write "操作规范"("" ("字符串")) -> ()
                    n580 = local write "new picture"(w1156) -> ()
                  }
                  frame True {
                    n581 = call <vilib>:"Read PNG File.vi"("path to PNG file"=path "Picture_Data/1.png" ("path to JPEG file")) -> ("image data"=w1161:T2)  [unwired: 8 in, 2 out]
                    n582 = call <vilib>:"Draw Flattened Pixmap.vi"("image data"=w1161) -> ("new picture"=w1157:picture)  [unwired: 8 in]
                    n583 = One Button Dialog(message="顶升油缸已就位，请引进新标准节！" ("消息")) -> ()  [unwired: 1 in, 1 out]
                    n584 = local write "操作规范"("顶升油缸已就位，请引进新标准节！" ("字符串")) -> ()
                    n585 = local write "new picture"(w1157) -> ()
                  }
                }
                n586 = case shown="真" w1094 {
                  frame False {
                    n587 = call "Empty Picture"() -> ("empty picture"=w1148:picture)
                    n588 = local write "new picture"(w1148) -> ()
                    n589 = local write "操作规范"("" ("字符串")) -> ()
                  }
                  frame True {
                    n590 = call <vilib>:"Read PNG File.vi"("path to PNG file"=path "Picture_Data/1.png" ("path to JPEG file")) -> ("image data"=w1154:T2)  [unwired: 8 in, 2 out]
                    n591 = call <vilib>:"Draw Flattened Pixmap.vi"("image data"=w1154) -> ("new picture"=w1150:picture)  [unwired: 8 in]
                    n592 = One Button Dialog(message="新标准节已引进，请压缩油缸！" ("消息")) -> ()  [unwired: 1 in, 1 out]
                    n593 = local write "操作规范"("新标准节已引进，请压缩油缸！" ("字符串")) -> ()
                    n594 = local write "new picture"(w1150) -> ()
                  }
                }
              }
              frame 170..180 {
                n595 = One Button Dialog(message="顶升冒顶警告！" ("消息")) -> ()  [unwired: 1 in, 1 out]
              }
              frame 110..115 {
                n596 = Equal?(x=w1175, y=1) -> (x = y?=w1202:bool)
                n597 = Equal?(x=w1174, y=1) -> (x = y?=w1203:bool)
                n598 = Equal?(x=w1164, y=0) -> (x = y?=w1213:bool)
                n599 = Equal?(x=w1163, y=1) -> (x = y?=w1214:bool)
                n600 = Equal?(x=w1165, y=0) -> (x = y?=w1212:bool)
                n601 = Equal?(x=w1167, y=0) -> (x = y?=w1210:bool)
                n602 = Equal?(x=w1173, y=0) -> (x = y?=w1204:bool)
                n603 = Equal?(x=w1168, y=0) -> (x = y?=w1209:bool)
                n604 = Equal?(x=w1170, y=0) -> (x = y?=w1207:bool)
                n605 = Equal?(x=w1171, y=0) -> (x = y?=w1206:bool)
                n606 = Equal?(x=w1169, y=0) -> (x = y?=w1208:bool)
                n607 = Equal?(x=w1166, y=0) -> (x = y?=w1211:bool)
                n608 = Equal?(x=w1172, y=0) -> (x = y?=w1205:bool)
                n609 = Compound Arithmetic op=AND ("复合运算")(w1202, w1203, w1204, w1205, w1206, w1207, w1208, w1209, w1210, w1211, w1212, w1213, w1214) -> (w1228:bool)
                n610 = Equal?(x=w1175, y=1) -> (x = y?=w1227:bool)
                n611 = Equal?(x=w1174, y=1) -> (x = y?=w1226:bool)
                n612 = Equal?(x=w1164, y=1) -> (x = y?=w1216:bool)
                n613 = Equal?(x=w1163, y=1) -> (x = y?=w1215:bool)
                n614 = Equal?(x=w1165, y=1) -> (x = y?=w1217:bool)
                n615 = Equal?(x=w1167, y=1) -> (x = y?=w1219:bool)
                n616 = Equal?(x=w1173, y=0) -> (x = y?=w1225:bool)
                n617 = Equal?(x=w1168, y=0) -> (x = y?=w1220:bool)
                n618 = Equal?(x=w1170, y=0) -> (x = y?=w1222:bool)
                n619 = Equal?(x=w1171, y=0) -> (x = y?=w1223:bool)
                n620 = Equal?(x=w1169, y=0) -> (x = y?=w1221:bool)
                n621 = Equal?(x=w1166, y=1) -> (x = y?=w1218:bool)
                n622 = Equal?(x=w1172, y=0) -> (x = y?=w1224:bool)
                n623 = Compound Arithmetic op=AND ("复合运算")(w1227, w1226, w1225, w1224, w1223, w1222, w1221, w1220, w1219, w1218, w1217, w1216, w1215) -> (w1229:bool)
                n624 = case shown="真" w1229 {
                  frame False {
                    n625 = call "Empty Picture"() -> ("empty picture"=w1230:picture)
                    n626 = local write "new picture"(w1230) -> ()
                    n627 = local write "操作规范"("" ("字符串")) -> ()
                  }
                  frame True {
                    n628 = call <vilib>:"Read PNG File.vi"("path to PNG file"=path "Picture_Data/1.png" ("path to JPEG file")) -> ("image data"=w1236:T2)  [unwired: 8 in, 2 out]
                    n629 = call <vilib>:"Draw Flattened Pixmap.vi"("image data"=w1236) -> ("new picture"=w1232:picture)  [unwired: 8 in]
                    n630 = One Button Dialog(message="标准节与塔身已连接，请压缩油缸！" ("消息")) -> ()  [unwired: 1 in, 1 out]
                    n631 = local write "new picture"(w1232) -> ()
                    n632 = local write "操作规范"("标准节与塔身已连接，请压缩油缸！" ("字符串")) -> ()
                  }
                }
                n633 = case shown="真" w1228 {
                  frame False {
                    n634 = call "Empty Picture"() -> ("empty picture"=w1237:picture)
                    n635 = local write "new picture"(w1237) -> ()
                    n636 = local write "操作规范"("" ("字符串")) -> ()
                  }
                  frame True {
                    n637 = call <vilib>:"Read PNG File.vi"("path to PNG file"=path "Picture_Data/1.png" ("path to JPEG file")) -> ("image data"=w1243:T2)  [unwired: 8 in, 2 out]
                    n638 = call <vilib>:"Draw Flattened Pixmap.vi"("image data"=w1243) -> ("new picture"=w1239:picture)  [unwired: 8 in]
                    n639 = One Button Dialog(message="油缸已就位，请连接引进节与塔身！" ("消息")) -> ()  [unwired: 1 in, 1 out]
                    n640 = local write "new picture"(w1239) -> ()
                    n641 = local write "操作规范"("油缸已就位，请连接引进节与塔身！" ("字符串")) -> ()
                  }
                }
              }
            }
            "data out" <- w569
          }
        }
        n642 = property on="数据输出" class="Str"("Text.Scroll Position"=inf) -> ()  [unwired: 2 in, 2 out]
      }
    }
    n643 = String Length(string=w30) -> (length=w65:i32)
    n644 = Not Equal To 0?(x=w65) -> (x != 0?=w64:bool)
    n645 = case shown="真" w64 {
      tunnel: w30 -> [_ w429]
      frame False {
      }
      frame True {
        n646 = local read "开始配平"() -> (w430:bool)
        n647 = local read "数据输出 2"() -> (w428:string)
        n648 = case shown="真" w430 {
          tunnel: w429 -> [_ w458]
          tunnel: w428 -> [_ w461]
          frame False {
          }
          frame True {
            n649 = Concatenate Strings(w461, "\n", w458) -> (→"数据输出 2":string)
            n650 = String Subset(string=w458, offset (0)=1 ("偏移量(0)"), length (rest)=3 ("长度（剩余）")) -> (substring=w449:string)
            "子字符串" <- w449
            n651 = String Subset(string=w458, offset (0)=11 ("偏移量(0)"), length (rest)=3 ("长度（剩余）")) -> (substring=w445:string)
            "子字符串 3" <- w445
            n652 = String Subset(string=w458, offset (0)=16 ("偏移量(0)"), length (rest)=3 ("长度（剩余）")) -> (substring=w443:string)
            "子字符串 4" <- w443
            n653 = String Subset(string=w458, offset (0)=6 ("偏移量(0)"), length (rest)=3 ("长度（剩余）")) -> (substring=w446:string)
            "子字符串 2" <- w446
            n654 = Fract/Exp String To Number(string=w449, offset=0 ("偏移量")) -> (number=w441:dbl)  [unwired: 2 in, 1 out]
            "超声波雷达1" <- w441
            "超声波雷达1" <- w441
            n655 = Fract/Exp String To Number(string=w446, offset=0 ("默认(0 I32)")) -> (number=w440:dbl)  [unwired: 2 in, 1 out]
            "超声波雷达2" <- w440
            "超声波雷达2" <- w440
            n656 = Fract/Exp String To Number(string=w445, offset=0 ("默认(0 I32)")) -> (number=w432:dbl)  [unwired: 2 in, 1 out]
            "?" <- w432
            "超声波雷达35" <- w432
            n657 = Fract/Exp String To Number(string=w443, offset=0 ("偏移量")) -> (number=w431:dbl)  [unwired: 2 in, 1 out]
            "超声波雷达4 6" <- w431
            "超声波雷达4" <- w431
            n658 = Subtract(x=w432, y=w431) -> (x-y=w433:dbl)
            n659 = Subtract(x=w441, y=w440) -> (x-y=w439:dbl)
            n660 = Absolute Value(x=w433) -> (abs(x)=w434:dbl)
            n661 = Absolute Value(x=w439) -> (abs(x)=w438:dbl)
            n662 = Less?(x=w434, y=10.0) -> ()  [unwired: 1 out]
            n663 = Less?(x=w438, y=10.0) -> (x < y?=→"配平指示1":bool)
          }
        }
        n664 = property on="数据输出" class="Str"("Text.Scroll Position"=inf) -> ()  [unwired: 2 in, 2 out]
      }
    }
    n665 = case shown="真" "清空" {
      frame False {
      }
      frame True {
        n666 = local write "数据输出"("" ("数据输出")) -> ()
      }
    }
    n667 = case shown="真" "清空 2" {
      frame False {
      }
      frame True {
        n668 = local write "数据输出 2"("" ("数据输出")) -> ()
      }
    }
    n669 = Greater Or Equal?(x=w24, y=5.0) -> (x >= y?=w23:bool)
    n670 = Greater Or Equal?(x=w22, y=5.0) -> (x >= y?=w21:bool)
    n671 = case shown="真" w23 {
      frame False {
      }
      frame True {
        n672 = call <vilib>:"Read PNG File.vi"("path to PNG file"=path "Picture_Data/1.png" ("path to JPEG file")) -> ("image data"=w184:T2)  [unwired: 8 in, 2 out]
        n673 = call <vilib>:"Draw Flattened Pixmap.vi"("image data"=w184) -> ("new picture"=→"new picture 2":picture)  [unwired: 8 in]
        n674 = One Button Dialog(message="警告！顶升套架y轴倾角过大，请立即停止升降节！" ("消息")) -> ()  [unwired: 1 in, 1 out]
      }
    }
    n675 = Greater Or Equal?(x=w18, y=3.0) -> (x >= y?=w16:bool)
    n676 = case shown="真" w16 {
      frame False {
      }
      frame True {
        n677 = call <vilib>:"Read PNG File.vi"("path to PNG file"=path "Picture_Data/1.png" ("path to JPEG file")) -> ("image data"=w176:T2)  [unwired: 8 in, 2 out]
        n678 = call <vilib>:"Draw Flattened Pixmap.vi"("image data"=w176) -> ("new picture"=→"new picture 4":picture)  [unwired: 8 in]
        n679 = One Button Dialog(message="警告！风速过大，请立即停止升降节！" ("消息")) -> ()  [unwired: 1 in, 1 out]
      }
    }
    n680 = case shown="真" w21 {
      frame False {
      }
      frame True {
        n681 = call <vilib>:"Read PNG File.vi"("path to PNG file"=path "Picture_Data/1.png" ("path to JPEG file")) -> ("image data"=w180:T2)  [unwired: 8 in, 2 out]
        n682 = call <vilib>:"Draw Flattened Pixmap.vi"("image data"=w180) -> ("new picture"=→"new picture 3":picture)  [unwired: 8 in]
        n683 = One Button Dialog(message="警告！顶升套架x轴倾角过大，请立即停止升降节！" ("消息")) -> ()  [unwired: 1 in, 1 out]
      }
    }
    n684 = Number To Fractional String(number=w24) -> (F-format string=w38:string)  [unwired: 3 in]
    n685 = Number To Fractional String(number=w22) -> (F-format string=w39:string)  [unwired: 3 in]
    n686 = Number To Fractional String(number=w18) -> (F-format string=w44:string)  [unwired: 3 in]
    n687 = Number To Fractional String(number=w48) -> (F-format string=w47:string)  [unwired: 3 in]
    n688 = Number To Fractional String(number=w41) -> (F-format string=w37:string)  [unwired: 3 in]
    n689 = Number To Fractional String(number=w40) -> (F-format string=w34:string)  [unwired: 3 in]
    n690 = call <vilib>:"Read PNG File.vi"("path to PNG file"=path "Picture_Data/jacking_beam.png" ("path to JPEG file")) -> ("image data"=w104:T2)  [unwired: 8 in, 2 out]
    n691 = call <vilib>:"Read PNG File.vi"("path to PNG file"=path "Picture_Data/stanard_section.png" ("path to JPEG file")) -> ("image data"=w26:T2)  [unwired: 8 in, 2 out]
    n692 = call <vilib>:"Read PNG File.vi"("path to PNG file"=path "Picture_Data/pin_shaft.png" ("path to JPEG file")) -> ("image data"=w99:T2)  [unwired: 8 in, 2 out]
    n693 = call <vilib>:"Draw Flattened Pixmap.vi"("image data"=w104) -> ("new picture"=→"jacking_beam":picture)  [unwired: 8 in]
    n694 = call <vilib>:"Draw Flattened Pixmap.vi"("image data"=w26) -> ("new picture"=→"stanard_section 2":picture)  [unwired: 8 in]
    n695 = call <vilib>:"Draw Flattened Pixmap.vi"("image data"=w99) -> ("new picture"=→"pin_shaft":picture)  [unwired: 8 in]
    n696 = Concatenate Strings("Device_ID:001,Jacking_frame_x_axis:", "lack_usb" ("字符串"), ",Jacking_frame_y_axis:" ("字符串"), "lack_usb" ("字符串"), ",Jacking_height:" ("字符串"), w47, ",Wind_Speed:" ("字符串"), w44, ",Tower_Crane_body_x_axis:" ("字符串"), w39, ",Tower_Crane_body_y_axis:" ("字符串"), w38, ",Amplitude_Length:" ("字符串"), w37, ",Rotation_Angle:" ("字符串"), w34, ",Photoelectric_Switch:" ("字符串"), w31, ",Radar:" ("字符串"), w30) -> (w53:string)
    n697 = UDP Write(address=w61, port or service name=u16 10000 ("端口或服务名称"), connection ID=w62, data in=w53, 8:w58) -> (error out=w56:errorcluster, 3:w57:refnum<k16>)  [unwired: 1 in]
    n698 = call <vilib>:"Read PNG File.vi"("path to PNG file"=path "Picture_Data/rotary_support.png" ("path to JPEG file")) -> ("image data"=w93:T2)  [unwired: 8 in, 2 out]
    n699 = call <vilib>:"Read PNG File.vi"("path to PNG file"=path "Picture_Data/stanard_section.png" ("path to JPEG file")) -> ("image data"=w98:T2)  [unwired: 8 in, 2 out]
    n700 = call <vilib>:"Draw Flattened Pixmap.vi"("image data"=w93) -> ("new picture"=→"rotary_support":picture)  [unwired: 8 in]
    n701 = call <vilib>:"Draw Flattened Pixmap.vi"("image data"=w98) -> ("new picture"=→"stanard_section":picture)  [unwired: 8 in]
    n702 = call <vilib>:"Read PNG File.vi"("path to PNG file"=path "Picture_Data/section_connect.png" ("path to JPEG file")) -> ("image data"=w90:T2)  [unwired: 8 in, 2 out]
    n703 = call <vilib>:"Draw Flattened Pixmap.vi"("image data"=w90) -> ("new picture"=→"section_connect":picture)  [unwired: 8 in]
  }
  n704 = UDP Close(connection ID=w12, 8:w13) -> ()  [unwired: 2 out]
  n705 = UDP Close(connection ID=w2, 8:w1) -> ()  [unwired: 2 out]
  n706 = UDP Close(connection ID=w8, 8:w6) -> ()  [unwired: 2 out]
